vi "laneleftright412.vi"() -> (2 "Coeff right":dbl[](array[numeric]), 3 "Coeff left":dbl[](array[numeric]))   [LabVIEW 2015]
uses:
  <vilib>/Analysis/polynomials.llb/Remove Zero Threshold Type.ctl
  <vilib>/Analysis/1siggen.llb/Ramp Pattern by Samples.vi
  G_SEN.vi
  <vilib>/Analysis/1siggen.llb/Ramp Pattern by Delta.vi
  G_ALL.vi
  G_LCM.vi
  <vilib>/Analysis/polynomials.llb/1D Polynomial Evaluation (DBL).vi
  <vilib>/Analysis/polynomials.llb/Remove Zero Coefficients (DBL).vi
  <vilib>/Analysis/NI_AALPro.lvlib
  <vilib>/Analysis/NI_AALBase.lvlib
  <vilib>/Analysis/6fits.llb/Curve Fitting Criteria.ctl
panel:
  out "point_flag":i32[](array[numeric])
  out "gap":dbl
  out "residue":dbl
  out "appended array":dbl[](array[numeric])
  out "Steering coeff":dbl[](array[numeric])
  out "Coeff stop 2":dbl[](array[numeric])
  out "min value":dbl
  out "rin":dbl[](array[numeric])
  out "rout":dbl[](array[numeric])
  out "r":dbl[](array[numeric])
  out "wgain":dbl[](array[numeric])
  out "y 2":dbl[](array[numeric])
  out "x 2":dbl[](array[numeric])
  out "w 2":dbl[](array[numeric])
  out "lane_right_pt":dbl[][](array[numeric])
  in  "x_gain":dbl=1.0 min=-1.0 max=1.0
  in  "y_gain":dbl=1.0 min=-1.0 max=1.0
  out "map_track 2":dbl[][](array[numeric])
  in  "d_safe":dbl=1.1 format="%#_13g"
  out "map_track":dbl[][](array[numeric])
  out "lane_left_pt":dbl[][](array[numeric])
  out "x_shift":dbl format="%#_13g"
  out "y_shift":dbl format="%#_13g"
  in  "lane_gain":dbl=0.7 min=-1.0 max=1.0
  out "Lane_C_M":dbl[](array[numeric])=[0.8601491478953653, 0.8717844136967624, 0.882947592858927, 0.8936326403234123, 0.9038337699485205, 0.9135454576426009, 0.9227624443554423, 0.9314797389261423, 0.9396926207859084, 0.9473966425143293, 0.9545876322477319, 0.9612616959383189, 0.9674152194628639, 0.9730448705798238, 0.9781476007338057, 0.9827206467064133, 0.9867615321125792, 0.9902680687415704, 0.993238357741943, 0.9956707906498045, 0.9975640502598242, 0.9989171113385246, 0.9997292411794617, 1.0, 0.9997292411794617, 0.9989171113385246, 0.9975640502598242, 0.9956707906498045, 0.993238357741943, 0.9902680687415704, 0.9867615321125792, 0.9827206467064133]
  out "ratio(-1:left1:right)":dbl
  out "NaN/Path/Refnum?":bool
  out "Rleft":dbl
  out "Rright":dbl
  out "poly":i32=2 min=1 max=5 step=1
  out "y_end":dbl[](array[numeric])=[0.8601491478953653, 0.8717844136967624, 0.882947592858927, 0.8936326403234123, 0.9038337699485205, 0.9135454576426009, 0.9227624443554423, 0.9314797389261423, 0.9396926207859084, 0.9473966425143293, 0.9545876322477319, 0.9612616959383189, 0.9674152194628639, 0.9730448705798238, 0.9781476007338057, 0.9827206467064133, 0.9867615321125792, 0.9902680687415704, 0.993238357741943, 0.9956707906498045, 0.9975640502598242, 0.9989171113385246, 0.9997292411794617, 1.0, 0.9997292411794617, 0.9989171113385246, 0.9975640502598242, 0.9956707906498045, 0.993238357741943, 0.9902680687415704, 0.9867615321125792, 0.9827206467064133]
  in  "iter":i32=2
  out "Waveform Graph":dbl[](graph)
  out "w":dbl[](array[numeric])
  out "XY Graph 4":cluster{"Y":dbl[], "Y":dbl[]}[](graph)=[{"Y"=array[3210 elements], "Y"=array[3210 elements]}, {"Y"=[-0.0, 0.001154394197769193, 0.004617650635850623, 0.010389990872226917, 0.018471784248973222, 0.02886354801042046, 0.041565947468740205, 0.056579796217107514, 0.0739060563904701, 0.0935458389742223, 0.11550040416098284, 0.13977116175580306, 0.16635967162997645, 0.19526764422393228, 0.2264969410994837, 0.26004957554195585, 0.2959277132125635, 0.3341336728515216, 0.374669927032528, 0.417539102969144, 0.4627439833735707, 0.5102875073687159, 0.560172771454063, 0.6124030305261954, 0.6669816989546717, 0.7239123517142048, 0.7831987255740245, 0.8448447203451934, 0.9088544001870815, 0.975231994973953, 1.0439819017227023, 1.1151086860829622, 1.1886170838907617, 1.2645120027869723, 1.342798523901962, 1.42348190360768, 1.5065675753387922, 1.592061151484188, 1.6799684253507792, 1.770295373200753, 1.8630481563645134, 1.9582331234307588, 2.0558568125157564, 2.1559259536137603, 2.258447471030621], "Y"=[0.0, 0.5, 1.0, 1.5, 2.0, 2.5, 3.0, 3.5, 4.0, 4.5, 5.0, 5.5, 6.0, 6.5, 7.0, 7.5, 8.0, 8.5, 9.0, 9.5, 10.0, 10.5, 11.0, 11.5, 12.0, 12.5, 13.0, 13.5, 14.0, 14.5, 15.0, 15.5, 16.0, 16.5, 17.0, 17.5, 18.0, 18.5, 19.0, 19.5, 20.0, 20.5, 21.0, 21.5, 22.0]}, {"Y"=[0.362252581831572], "Y"=[-0.8199241909738847]}, {"Y"=array[210 elements], "Y"=array[210 elements]}, {"Y"=[-0.925, -0.925, -0.925, -0.6775, -0.6775, -0.925, -0.925, -0.925, -0.925, -0.6775, -0.6775, -0.925, -0.925, -0.925, 0.9025, 0.9025, 0.9025, 0.6775, 0.6775, 0.9025, 0.9025, 0.9025, 0.9025, 0.6775, 0.6775, 0.9025, 0.9025, 0.9025, -0.925], "Y"=[-0.75, -0.224, 0.224, 0.224, -0.224, -0.224, 0.224, 2.415, 2.885, 2.885, 2.415, 2.415, 2.885, 3.5, 3.5, 2.885, 2.415, 2.415, 2.885, 2.885, 2.415, 0.224, -0.224, -0.224, 0.224, 0.224, -0.224, -0.75, -0.75]}, {"Y"=[0.171875, 0.15377271904051304, 0.1346290179491043, 0.11445423440635205, 0.09325870609283447, 0.07105277068912982, 0.04784676587581635, 0.02365102933347224, -0.0015241012573242174, -0.02766828821599482, -0.05477119386196136, -0.08282248051464558, -0.11181181049346922, -0.14172884611785413, -0.17256324970722198, -0.20430468358099463, -0.23694281005859374, -0.27046729145944115, -0.30486779010295867, -0.340133968308568, -0.3762554883956909, -0.41322201268374914, -0.4510232034921646, -0.4896487231403589], "Y"=[0.0, 0.5, 1.0, 1.5, 2.0, 2.5, 3.0, 3.5, 4.0, 4.5, 5.0, 5.5, 6.0, 6.5, 7.0, 7.5, 8.0, 8.5, 9.0, 9.5, 10.0, 10.5, 11.0, 11.5]}, {"Y"=[1.796875, 1.778772719040513, 1.7596290179491043, 1.739454234406352, 1.7182587060928345, 1.6960527706891297, 1.6728467658758164, 1.6486510293334722, 1.6234758987426758, 1.5973317117840051, 1.5702288061380387, 1.5421775194853544, 1.513188189506531, 1.483271153882146, 1.452436750292778, 1.4206953164190055, 1.3880571899414063, 1.354532708540559, 1.3201322098970414, 1.284866031691432, 1.248744511604309, 1.2117779873162509, 1.1739767965078354, 1.135351276859641, 1.0959117660522462, 1.0556686017662287, 1.014632121682167, 0.9728126634806396, 0.9302205648422242, 0.8868661634474992], "Y"=[0.0, 0.5, 1.0, 1.5, 2.0, 2.5, 3.0, 3.5, 4.0, 4.5, 5.0, 5.5, 6.0, 6.5, 7.0, 7.5, 8.0, 8.5, 9.0, 9.5, 10.0, 10.5, 11.0, 11.5, 12.0, 12.5, 13.0, 13.5, 14.0, 14.5]}, {"Y"=[-1.453125, -1.471227280959487, -1.4903709820508957, -1.510545765593648, -1.5317412939071655, -1.5539472293108703, -1.5771532341241836, -1.6013489706665278, -1.6265241012573242, -1.6526682882159949, -1.6797711938619613, -1.7078224805146456, -1.736811810493469, -1.766728846117854, -1.797563249707222, -1.8293046835809945, -1.8619428100585937, -1.895467291459441, -1.9298677901029586], "Y"=[0.0, 0.5, 1.0, 1.5, 2.0, 2.5, 3.0, 3.5, 4.0, 4.5, 5.0, 5.5, 6.0, 6.5, 7.0, 7.5, 8.0, 8.5, 9.0]}, {"Y"=[0.171875, 0.2568230007600336, 0.3384052130063493, 0.44574342526006827, 0.5205081969556753, 0.5917680690742042, 0.659409530134929, 0.7229937549325056, 0.7835496148685115, 0.8405449546633443, 0.9258576868463875], "Y"=[-20.239964538708662, -19.725637940364884, -19.211158961966362, -18.6998967366845, -18.19022720070031, -17.681887266143153, -17.17615515566314, -16.67683575591291, -16.176265245349786, -15.679082775270938, -15.183754484614711]}, {"Y"=[7.134647485270904], "Y"=[38.71960961082238]}, {"Y"=array[980 elements], "Y"=array[980 elements]}, {"Y"=[], "Y"=[]}]
  out "y":dbl[](array[numeric])
  out "x":dbl[](array[numeric])
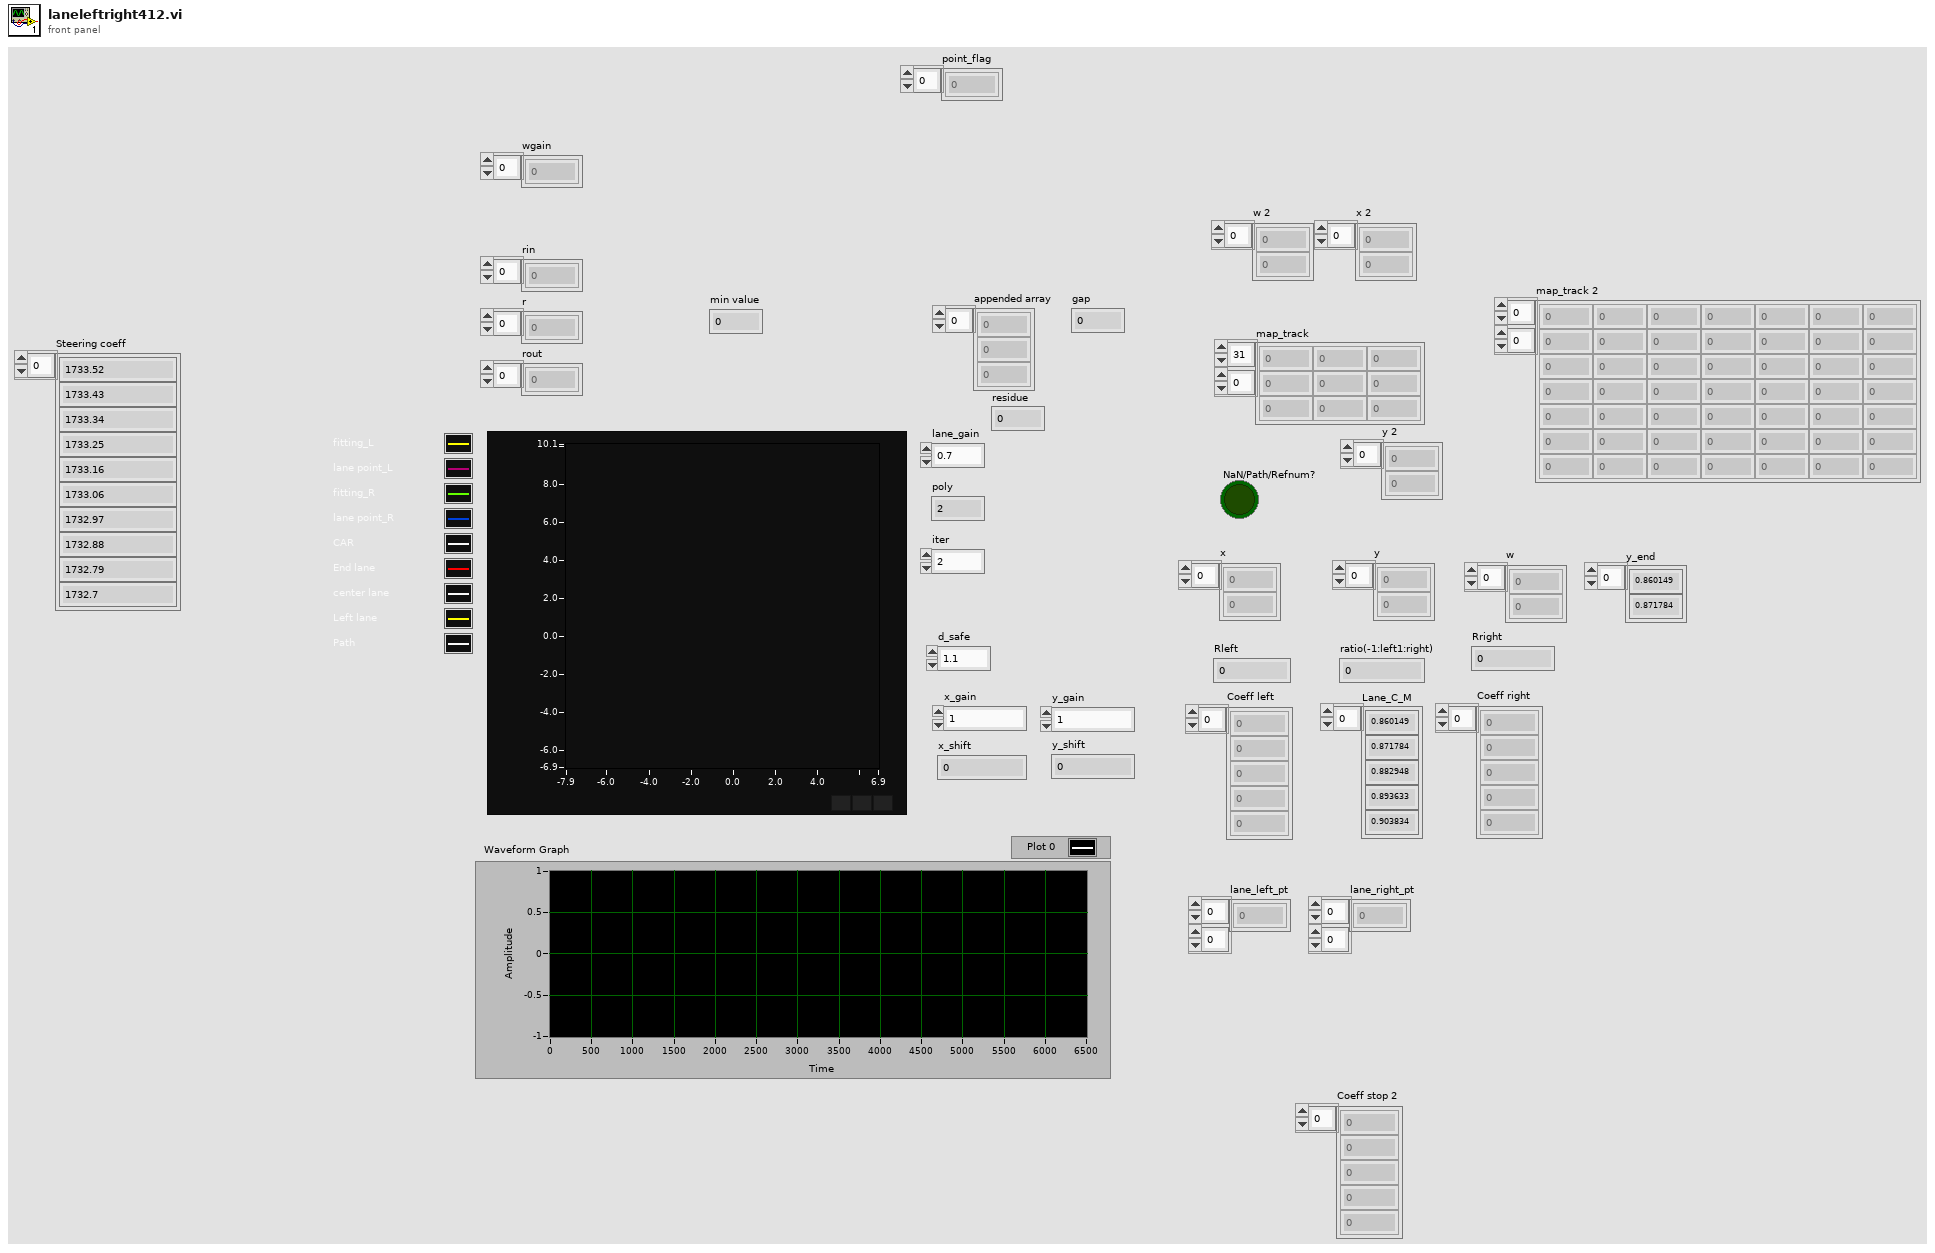
[diagram p1: front panel]
types:
  T1 = cluster{"C_Wheel base":dbl, "ratio_steer":dbl, "Overall width":dbl, "af":dbl, "turn radius":dbl, "eval":dbl, "ap":dbl, "an":dbl, "Vmax":dbl, "mu":dbl, "Vlast":dbl}
  T2 = cluster{"hash":i64, "sys time":i64, "size":i64, "x":dbl[], "y":dbl[], "point_flag":i32[]}
  T3 = cluster{"delta":bool, "Rotational position":dbl, "Rotational position":dbl, "Numeric":i32}[]
  T4 = cluster{"Steer_input":dbl, "Steer_output":dbl, "VS_des":dbl, "VS_can":dbl, "heading":dbl, "auto":bool, "run":bool, "x":dbl, "y":dbl, "slam_y":dbl, "slam_x":dbl, "slam_heading":dbl}
  T5 = typedef "NI_AALPro.lvlib/Curve Fitting Criteria.ctl" = u16
  T6 = typedef "NI_AALPro.lvlib/Remove Zero Threshold Type.ctl" = u16
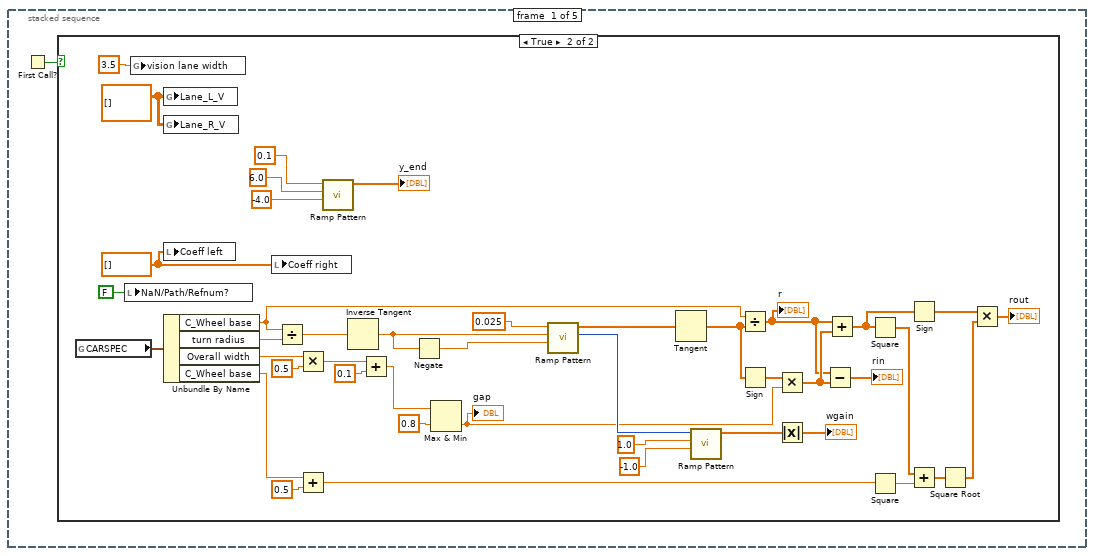
[diagram p2: hidden frame]
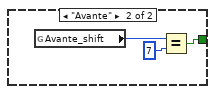
[diagram p5: hidden frame]
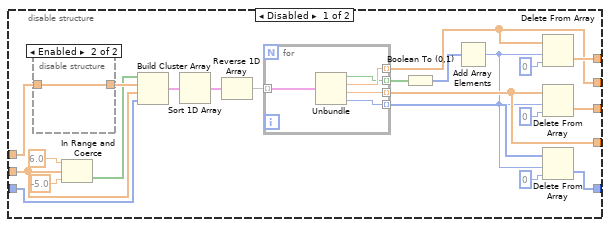
[diagram p6: hidden frame]
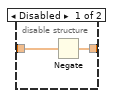
[diagram p7: hidden frame]
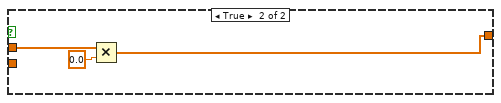
[diagram p8: hidden frame]
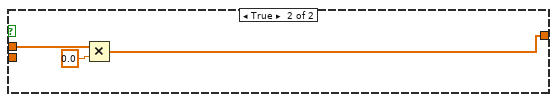
[diagram p9: hidden frame]
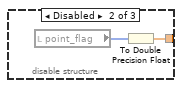
[diagram p10: hidden frame]
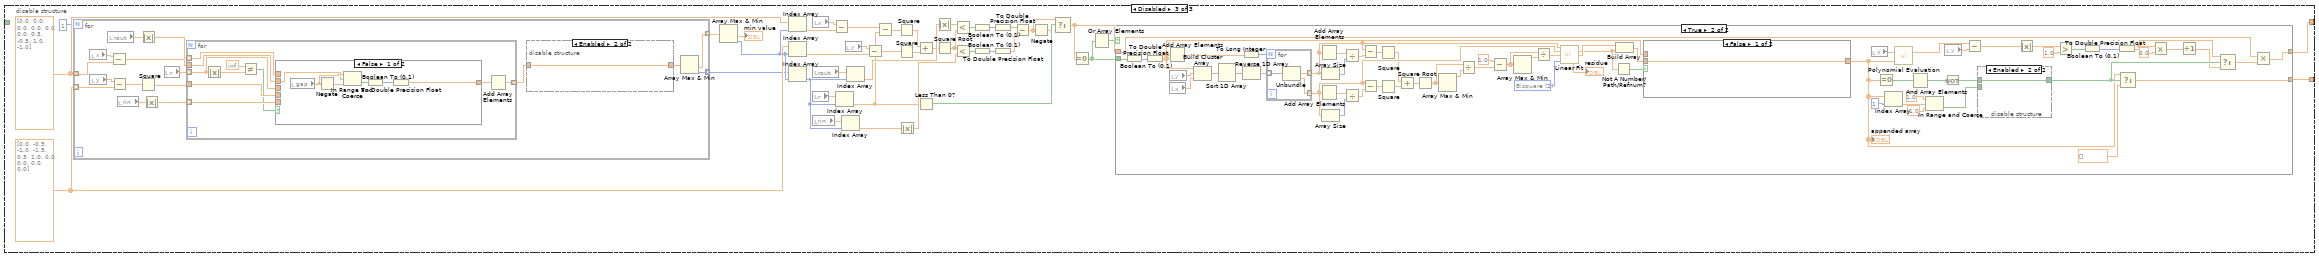
[diagram p11: hidden frame]
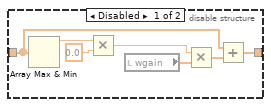
[diagram p12: hidden frame]
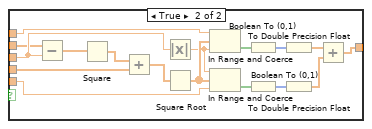
[diagram p13: hidden frame]
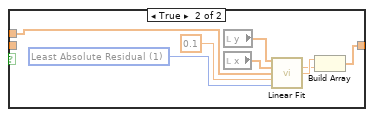
[diagram p15: hidden frame]
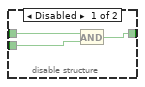
[diagram p16: hidden frame]
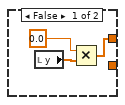
[diagram p17: hidden frame]
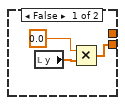
[diagram p18: hidden frame]
diagram:
  n1 = stacked-sequence {
    frame #0 {
      n2 = First Call?() -> (First Call?: T/F=w1:bool)
      n3 = case shown="True" w1 {
        frame False {
        }
        frame True {
          w37 = dbl[] [] ("Coeff left")
          w39 = dbl[][] [] ("Lane_R_V")
          n4 = global read "G_ALL.vi" "CARSPEC"() -> (w10:T1)
          n5 = local write "NaN/Path/Refnum?"(FALSE ("NaN/Path/Refnum?")) -> ()
          n6 = global write "G_SEN.vi" "vision lane width"(3.5 ("vision lane width")) -> ()
          n7 = global write "G_SEN.vi" "Lane_L_V"(w39) -> ()
          n8 = global write "G_SEN.vi" "Lane_R_V"(w39) -> ()
          n9 = local write "Coeff left"(w37) -> ()
          n10 = Unbundle By Name(w10) -> ("C_Wheel base"=w17:dbl, "turn radius"=w11:dbl, "Overall width"=w18:dbl, "C_Wheel base"=w3:dbl)
          n11 = local write "Coeff right"(w37) -> ()
          n12 = Divide(x=w17, y=w11) -> (x/y=w12:dbl)
          n13 = Multiply(x=w18, y=0.5) -> (x*y=w9:dbl)
          n14 = Add(x=w3, y=0.5) -> (x+y=w2:dbl)
          n15 = call-poly <vilib>:"Ramp Pattern.vi"("start"=-4.0, "end"=6.0, "delta"=0.1) -> ("Ramp Pattern"=→"y_end":dbl[])  [unwired: 6 in, 2 out]
          n16 = Inverse Tangent(1:w12) -> (0:w14:dbl)
          n17 = Add(x=w9, y=0.1) -> (x+y=w6:dbl)
          n18 = Negate(x=w14) -> (-x=w13:dbl)
          n19 = Max & Min(x=w6, y=0.8) -> (min(x,y)=w5:dbl)  [unwired: 1 out]
          "gap" <- w5
          n20 = call-poly <vilib>:"Ramp Pattern.vi"("start"=w13, "end"=w14, "delta"=0.025) -> ("samples"=w32:i32, "Ramp Pattern"=w16:dbl[])  [unwired: 6 in, 1 out]
          n21 = Tangent(1:w16) -> (0:w20:dbl[])
          n22 = call-poly <vilib>:"Ramp Pattern.vi"("start"=-1.0, "end"=1.0, "samples"=w32) -> ("Ramp Pattern"=w35:dbl[])  [unwired: 7 in, 1 out]
          n23 = Divide(x=w17, y=w20) -> (x/y=w23:dbl[])
          "r" <- w23
          n24 = Sign(1:w20) -> (0:w21:dbl[])
          n25 = Multiply(x=w21, y=w5) -> (x*y=w24:dbl[])
          n26 = Absolute Value(x=w35) -> (abs(x)=→"wgain":dbl[])
          n27 = Subtract(x=w23, y=w24) -> (x-y=→"rin":dbl[])
          n28 = Add(x=w23, y=w24) -> (x+y=w28:dbl[])
          n29 = Square(x=w28) -> (x^2=w25:dbl[])
          n30 = Square(x=w2) -> (x^2=w26:dbl)
          n31 = Sign(1:w28) -> (0:w30:dbl[])
          n32 = Add(x=w25, y=w26) -> (x+y=w27:dbl[])
          n33 = Square Root(x=w27) -> (sqrt(x)=w29:dbl[])
          n34 = Multiply(x=w30, y=w29) -> (x*y=→"rout":dbl[])
        }
      }
    }
    frame #1 {
      n35 = flat-sequence {
        tunnel: [w48] -> w45
        tunnel: w45 -> [w97]
        frame #0 {
          n36 = global read "G_LCM.vi" "VISION_LANE_PT"() -> (w52:T2)
          n37 = Unbundle By Name(w52) -> ("x"=w56:dbl[], "y"=w53:dbl[], "point_flag"=w46:i32[])
          n38 = disable-structure shown="Enabled" {
            disable-tunnel: w56 -> [w83 w95]
            disable-tunnel: [w81 w94] -> w55
            disable-tunnel: [w80 w95] -> w54
            disable-tunnel: w53 -> [w78 w94]
            disable-tunnel: [w69 w95] -> w51
            disable-tunnel: [w68 w94] -> w50
            disable-tunnel: [w63 w93] -> w47
            disable-tunnel: w46 -> [w67 w93]
            frame Disabled {
              n39 = disable-structure shown="Enabled" {
                disable-tunnel: w83 -> [w86 w87]
                disable-tunnel: [w85 w87] -> w84
                frame Disabled {
                  n40 = Negate(x=w86) -> (-x=w85:dbl[])
                }
                frame Enabled {
                }
              }
              n41 = In Range and Coerce(upper limit=6.0 ("delta"), x=w78, lower limit=-5.0) -> (In Range?=w76:bool[])  [unwired: 1 out]
              n42 = Build Cluster Array(w76, w84, w78, w67) -> (w74:T3)
              n43 = Sort 1D Array(array=w74) -> (sorted array=w75:T3)
              n44 = Reverse 1D Array(array=w75) -> (reversed array=w71:T3)
              n45 = for {
                tunnel: w71 -> [w92] mode=indexing
                tunnel: [w91] -> w69 mode=indexing
                tunnel: [w90] -> w68 mode=indexing
                tunnel: [w89] -> w79 mode=indexing
                tunnel: [w88] -> w66 mode=indexing
                n46 = Unbundle(w92) -> ("delta"=w89:bool, "Rotational position"=w91:dbl, "Rotational position"=w90:dbl, "Numeric"=w88:i32)
              }
              n47 = Boolean To (0,1)(Boolean=w79) -> (0, 1=w72:i16[])
              n48 = Add Array Elements(numeric array=w72) -> (sum=w65:i16)
              n49 = Delete From Array(array=w69, length=w65, index=0) -> (deleted portion=w80:dbl[])  [unwired: 1 out]
              n50 = Delete From Array(array=w68, length=w65, index=0) -> (deleted portion=w81:dbl[])  [unwired: 1 out]
              n51 = Delete From Array(array=w66, length=w65, index=0) -> (deleted portion=w63:i32[])  [unwired: 1 out]
            }
            frame Enabled {
            }
          }
          "x" <- w54
          "y" <- w55
          "x 2" <- w51
          "y 2" <- w50
          "point_flag" <- w47
          n52 = global read "G_LCM.vi" "car name"() -> (w49:string)
          n53 = case shown="Default" w49 {
            tunnel: [w57 w60] -> w48
            frame Default {
              n54 = global read "G_ALL.vi" "CARDATA"() -> (w59:T4)
              n55 = Unbundle By Name(w59) -> ("VS_can"=w58:dbl)
              n56 = Less Than 0?(x=w58) -> (x < 0?=w57:bool)
            }
            frame "Avante" {
              n57 = global read "G_ALL.vi" "Avante_shift"() -> (w62:u8)
              n58 = Equal?(x=w62, y=u8 7) -> (x = y?=w60:bool)
            }
          }
        }
        frame #1 {
          n59 = disable-structure shown="Enabled" {
            disable-tunnel: [w101 w163 w205] -> w96
            disable-tunnel: [_ _ w204] -> w98
            disable-tunnel: w97 -> [_ _ _]
            frame Enabled {
              n60 = local read "Coeff left"() -> (w130:dbl[])
              n61 = local read "Coeff right"() -> (w129:dbl[])
              n62 = Empty Array?(array=w130) -> (empty?=w131:bool)
              n63 = Empty Array?(array=w129) -> (empty?=w132:bool)
              n64 = local read "y"() -> (w127:dbl[])
              n65 = local read "x"() -> (w99:dbl[])
              n66 = local read "y"() -> (w133:dbl[])
              n67 = case shown="False" w131 {
                tunnel: w127 -> [w153 w161]
                tunnel: w130 -> [w150 _]
                tunnel: [w148 w160] -> w128
                frame False {
                  n68 = call-poly <vilib>:"Polynomial Evaluation.vi"("P(x)"=w150, "A"=w153) -> ("P(A)"=w152:dbl[])  [unwired: 1 out]
                  n69 = local read "x"() -> (w151:dbl[])
                  n70 = Subtract(x=w152, y=w151) -> (x-y=w157:dbl[])
                  n71 = Absolute Value(x=w157) -> (abs(x)=w156:dbl[])
                  n72 = Negate(x=w156) -> (-x=w155:dbl[])
                  n73 = Add(x=w155, y=1.0) -> (x+y=w159:dbl[])
                  n74 = Max & Min(x=0.0, y=w159) -> (max(x,y)=w149:dbl[])  [unwired: 1 out]
                  n75 = Negate(x=w149) -> (-x=w148:dbl[])
                }
                frame True {
                  n76 = Multiply(x=w161, y=0.0) -> (x*y=w160:dbl[])
                }
              }
              n77 = local read "y"() -> (w100:dbl[])
              n78 = case shown="False" w132 {
                tunnel: [w142 w145] -> w125
                tunnel: w129 -> [w141 _]
                tunnel: w133 -> [w134 w146]
                frame False {
                  n79 = call-poly <vilib>:"Polynomial Evaluation.vi"("P(x)"=w141, "A"=w134) -> ("P(A)"=w139:dbl[])  [unwired: 1 out]
                  n80 = local read "x"() -> (w140:dbl[])
                  n81 = Subtract(x=w139, y=w140) -> (x-y=w135:dbl[])
                  n82 = Absolute Value(x=w135) -> (abs(x)=w136:dbl[])
                  n83 = Negate(x=w136) -> (-x=w137:dbl[])
                  n84 = Add(x=w137, y=1.0) -> (x+y=w143:dbl[])
                  n85 = Max & Min(x=0.0, y=w143) -> (max(x,y)=w142:dbl[])  [unwired: 1 out]
                }
                frame True {
                  n86 = Multiply(x=w146, y=0.0) -> (x*y=w145:dbl[])
                }
              }
              n87 = Subtract(x=w99, y=6.0) -> (x-y=w103:dbl[])
              n88 = Subtract(x=w100, y=0.0) -> (x-y=w112:dbl[])
              n89 = Subtract(x=w99, y=-6.0) -> (x-y=w105:dbl[])
              n90 = Square(x=w105) -> (x^2=w104:dbl[])
              n91 = Square(x=w103) -> (x^2=w113:dbl[])
              n92 = Square(x=w112) -> (x^2=w114:dbl[])
              n93 = Add(x=w104, y=w114) -> (x+y=w120:dbl[])
              n94 = Add(x=w114, y=w113) -> (x+y=w115:dbl[])
              n95 = In Range and Coerce(upper limit=36.0, x=w120, lower limit=4.0) -> (In Range?=w122:bool[])  [unwired: 1 out]
              n96 = In Range and Coerce(upper limit=36.0, x=w115, lower limit=4.0) -> (In Range?=w121:bool[])  [unwired: 1 out]
              n97 = Boolean To (0,1)(Boolean=w122) -> (0, 1=w123:i16[])
              n98 = Boolean To (0,1)(Boolean=w121) -> (0, 1=w124:i16[])
              n99 = Multiply(x=i16 -1, y=w123) -> (x*y=w108:i16[])
              n100 = Add(x=w108, y=w124) -> (x+y=w110:i16[])
              n101 = Multiply(x=w110, y=1.0 ("element")) -> (x*y=w126:dbl[])
              n102 = Compound Arithmetic op=ADD(w126, w125, w128) -> (w101:dbl[])
            }
            frame Disabled {
              n103 = local read "point_flag"() -> (w164:i32[])
              n104 = To Double Precision Float(number=w164) -> (double precision float=w163:dbl[])
            }
            frame Disabled {
              w171 = dbl[] [0.0, -0.5, -1.0, -1.5, 0.5, 1.0, 0.0, 0.0, 0.0, 0.0]
              w169 = dbl[] [0.0, 0.0, 0.0, 0.0, 0.0, 0.0, 0.5, -0.5, 1.0, -1.0]
              n105 = for {
                N: 1 -> [_]
                tunnel: [w206] -> w166 mode=indexing
                tunnel: w169 -> [w211] mode=indexing
                tunnel: w171 -> [w209] mode=indexing
                tunnel: [w208] -> w167 mode=indexing
                n106 = local read "x"() -> (w213:dbl[])
                n107 = local read "y"() -> (w210:dbl[])
                n108 = local read "rout"() -> (w219:dbl[])
                n109 = Subtract(x=w213, y=w211) -> (x-y=w212:dbl[])
                n110 = Subtract(x=w210, y=w209) -> (x-y=w207:dbl[])
                n111 = local read "rin"() -> (w217:dbl[])
                n112 = Square(x=w207) -> (x^2=w220:dbl[])
                n113 = Absolute Value(x=w219) -> (abs(x)=w218:dbl[])
                n114 = Absolute Value(x=w217) -> (abs(x)=w216:dbl[])
                n115 = local read "r"() -> (w221:dbl[])
                n116 = for {
                  tunnel: w221 -> [w231] mode=indexing
                  tunnel: w220 -> [w239]
                  tunnel: w218 -> [w238] mode=indexing
                  tunnel: w216 -> [w237] mode=indexing
                  tunnel: [w236] -> w214 mode=indexing
                  tunnel: w212 -> [w235]
                  n117 = Absolute Value(x=w231) -> (abs(x)=w233:dbl)
                  n118 = Not Equal?(x=inf, y=w233) -> (x != y?=w230:bool)
                  n119 = case shown="False" w230 {
                    tunnel: w239 -> [_ w260]
                    tunnel: w238 -> [_ w257]
                    tunnel: w237 -> [_ w256]
                    tunnel: w231 -> [_ w252]
                    tunnel: w235 -> [w241 w247]
                    tunnel: [w240 w246] -> w234
                    frame False {
                      n120 = local read "gap"() -> (w242:dbl)
                      n121 = Negate(x=w242) -> (-x=w243:dbl)
                      n122 = In Range and Coerce(upper limit=w242, x=w241, lower limit=w243) -> (In Range?=w245:bool[])  [unwired: 1 out]
                      n123 = Boolean To (0,1)(Boolean=w245) -> (0, 1=w244:i16[])
                      n124 = To Double Precision Float(number=w244) -> (double precision float=w240:dbl[])
                    }
                    frame True {
                      n125 = Subtract(x=w247, y=w252) -> (x-y=w262:dbl[])
                      n126 = Square(x=w262) -> (x^2=w261:dbl[])
                      n127 = Add(x=w261, y=w260) -> (x+y=w259:dbl[])
                      n128 = Absolute Value(x=w252) -> (abs(x)=w253:dbl)
                      n129 = Square Root(x=w259) -> (sqrt(x)=w258:dbl[])
                      n130 = In Range and Coerce(upper limit=w257, x=w258, lower limit=w253) -> (In Range?=w249:bool[])  [unwired: 1 out]
                      n131 = In Range and Coerce(upper limit=w253, x=w258, lower limit=w256) -> (In Range?=w248:bool[])  [unwired: 1 out]
                      n132 = Boolean To (0,1)(Boolean=w249) -> (0, 1=w255:i16[])
                      n133 = Boolean To (0,1)(Boolean=w248) -> (0, 1=w254:i16[])
                      n134 = To Double Precision Float(number=w255) -> (double precision float=w251:dbl[])
                      n135 = To Double Precision Float(number=w254) -> (double precision float=w250:dbl[])
                      n136 = Add(x=w251, y=w250) -> (x+y=w246:dbl[])
                    }
                  }
                  n137 = Add Array Elements(numeric array=w234) -> (sum=w236:dbl)
                }
                n138 = disable-structure shown="Enabled" {
                  disable-tunnel: [w228 w229] -> w215
                  disable-tunnel: w214 -> [w224 w229]
                  frame Disabled {
                    n139 = Array Max & Min(array=w224) -> (max value=w227:dbl)  [unwired: 3 out]
                    n140 = Multiply(x=w227, y=0.0) -> (x*y=w223:dbl)
                    n141 = local read "wgain"() -> (w222:dbl[])
                    n142 = Multiply(x=w223, y=w222) -> (x*y=w225:dbl[])
                    n143 = Add(x=w224, y=w225) -> (x+y=w228:dbl[])
                  }
                  frame Enabled {
                  }
                }
                n144 = Array Max & Min(array=w215) -> (min value=w206:dbl, min index (indices)=w208:i32)  [unwired: 2 out]
              }
              n145 = Array Max & Min(array=w166) -> (min value=→"min value":dbl, min index (indices)=w170:i32)  [unwired: 2 out]
              n146 = Index Array(array=w169, index=w170) -> (element=w173:dbl)
              n147 = Index Array(array=w171, index=w170) -> (element=w172:dbl)
              n148 = Index Array(array=w167, index=w170) -> (element=w174:i32)
              n149 = local read "x"() -> (w197:dbl[])
              n150 = local read "rout"() -> (w193:dbl[])
              n151 = local read "r"() -> (w191:dbl[])
              n152 = local read "rin"() -> (w186:dbl[])
              n153 = Subtract(x=w197, y=w173) -> (x-y=w198:dbl[])
              n154 = Index Array(array=w191, index=w174) -> (element=w178:dbl)
              n155 = Index Array(array=w186, index=w174) -> (element=w180:dbl)
              n156 = local read "y"() -> (w199:dbl[])
              n157 = Index Array(array=w193, index=w174) -> (element=w192:dbl)
              n158 = Subtract(x=w199, y=w172) -> (x-y=w200:dbl[])
              n159 = Subtract(x=w198, y=w178) -> (x-y=w190:dbl[])
              n160 = Square(x=w190) -> (x^2=w189:dbl[])
              n161 = Square(x=w200) -> (x^2=w188:dbl[])
              n162 = Absolute Value(x=w180) -> (abs(x)=w179:dbl)
              n163 = Add(x=w189, y=w188) -> (x+y=w187:dbl[])
              n164 = Less Than 0?(x=w178) -> (x < 0?=w177:bool)
              n165 = Absolute Value(x=w192) -> (abs(x)=w194:dbl)
              n166 = Square Root(x=w187) -> (sqrt(x)=w195:dbl[])
              n167 = Less?(x=w194, y=w195) -> (x < y?=w196:bool[])
              n168 = Less?(x=w195, y=w179) -> (x < y?=w185:bool[])
              n169 = Boolean To (0,1)(Boolean=w196) -> (0, 1=w182:i16[])
              n170 = Boolean To (0,1)(Boolean=w185) -> (0, 1=w184:i16[])
              n171 = To Double Precision Float(number=w182) -> (double precision float=w181:dbl[])
              n172 = To Double Precision Float(number=w184) -> (double precision float=w183:dbl[])
              n173 = Subtract(x=w181, y=w183) -> (x-y=w176:dbl[])
              n174 = Negate(x=w176) -> (-x=w175:dbl[])
              n175 = Select(t=w176, s=w177, f=w175) -> (s? t:f=w203:dbl[])
              n176 = Equal To 0?(x=w203) -> (x = 0?=w202:bool[])
              n177 = Or Array Elements(Boolean array=w202) -> (logical OR=w201:bool)
              n178 = case shown="True" w201 {
                tunnel: [w263 w306] -> w205
                tunnel: w203 -> [w263 w305]
                tunnel: w202 -> [_ w298]
                tunnel: [_ w297] -> w204
                frame False {
                }
                frame True {
                  w299 = T5 2 items=["Least Square", "Least Absolute Residual", "Bisquare"] ("method")
                  n179 = Boolean To (0,1)(Boolean=w298) -> (0, 1=w302:i16[])
                  n180 = To Double Precision Float(number=w302) -> (double precision float=w289:dbl[])
                  n181 = Add Array Elements(numeric array=w289) -> (sum=w288:dbl)
                  n182 = local read "y"() -> (w293:dbl[])
                  n183 = local read "x"() -> (w292:dbl[])
                  n184 = Build Cluster Array(w289, w293, w292) -> (w291:cluster{dbl, dbl, dbl}[])
                  n185 = Sort 1D Array(array=w291) -> (sorted array=w290:cluster{dbl, dbl, dbl}[])
                  n186 = To Long Integer(number=w288) -> (32bit integer=w287:i32)
                  n187 = Reverse 1D Array(array=w290) -> (reversed array=w286:cluster{dbl, dbl, dbl}[])
                  n188 = for {
                    N: w287 -> [_]
                    tunnel: w286 -> [w329] mode=indexing
                    tunnel: [w328] -> w278 mode=indexing
                    tunnel: [w327] -> w276 mode=indexing
                    n189 = Unbundle(w329) -> (w328:dbl, w327:dbl)  [unwired: 1 out]
                  }
                  n190 = Add Array Elements(numeric array=w278) -> (sum=w282:dbl)
                  n191 = Add Array Elements(numeric array=w276) -> (sum=w281:dbl)
                  n192 = Array Size(array=w278) -> (size(s)=w283:i32)
                  n193 = Array Size(array=w276) -> (size(s)=w280:i32)
                  n194 = Divide(x=w282, y=w283) -> (x/y=w279:dbl)
                  n195 = Divide(x=w281, y=w280) -> (x/y=w277:dbl)
                  n196 = Subtract(x=w278, y=w279) -> (x-y=w275:dbl[])
                  n197 = Subtract(x=w276, y=w277) -> (x-y=w274:dbl[])
                  n198 = Square(x=w275) -> (x^2=w272:dbl[])
                  n199 = Square(x=w274) -> (x^2=w273:dbl[])
                  n200 = Add(x=w272, y=w273) -> (x+y=w271:dbl[])
                  n201 = Square Root(x=w271) -> (sqrt(x)=w269:dbl[])
                  n202 = Array Max & Min(array=w269) -> (max value=w270:dbl)  [unwired: 3 out]
                  n203 = Divide(x=w269, y=w270) -> (x/y=w268:dbl[])
                  n204 = Subtract(x=1.0, y=w268) -> (x-y=w265:dbl[])
                  n205 = Array Max & Min(array=w265) -> (max value=w266:dbl)  [unwired: 3 out]
                  n206 = Divide(x=w265, y=w266) -> (x/y=w264:dbl[])
                  n207 = call <vilib>:"Linear Fit.vi"("Y"=w278, "X"=w276, "Weight"=w264, "method"=w299) -> ("slope"=w296:dbl, "intercept"=w300:dbl, "residue"=→"residue":dbl)  [unwired: 7 in, 2 out]
                  n208 = Not A Number/Path/Refnum?(number/path/refnum=w296) -> (NaN/Path/Refnum?=w285:bool)
                  n209 = Build Array(w300, w296) -> (w294:dbl[])
                  n210 = case shown="False" w285 {
                    tunnel: w289 -> [_ w336]
                    tunnel: [w330 w333] -> w295
                    tunnel: w294 -> [w330 _]
                    frame False {
                    }
                    frame True {
                      w338 = T5 1 items=["Least Square", "Least Absolute Residual", "Bisquare"] ("method")
                      n211 = local read "y"() -> (w332:dbl[])
                      n212 = local read "x"() -> (w331:dbl[])
                      n213 = call <vilib>:"Linear Fit.vi"("Y"=w332, "X"=w331, "Weight"=w336, "tolerance"=0.1, "method"=w338) -> ("slope"=w334:dbl, "intercept"=w335:dbl)  [unwired: 6 in, 3 out]
                      n214 = Build Array(w335, w334) -> (w333:dbl[])
                    }
                  }
                  "appended array" <- w295
                  n215 = local read "x"() -> (w307:dbl[])
                  n216 = Equal To 0?(x=w295) -> (x = 0?=w321:bool[])
                  n217 = Index Array(array=w295, index=1) -> (element=w314:dbl)
                  n218 = call-poly <vilib>:"Polynomial Evaluation.vi"("P(x)"=w295, "A"=w307) -> ("P(A)"=w308:dbl[])  [unwired: 1 out]
                  n219 = And Array Elements(Boolean array=w321) -> (logical AND=w324:bool)
                  n220 = In Range and Coerce(upper limit=1.0, x=w314, lower limit=-1.0) -> (In Range?=w322:bool)  [unwired: 1 out]
                  n221 = Not(x=w324) -> (.not. x?=w325:bool)
                  n222 = local read "y"() -> (w309:dbl[])
                  n223 = Subtract(x=w308, y=w309) -> (x-y=w301:dbl[])
                  n224 = disable-structure shown="Enabled" {
                    disable-tunnel: w322 -> [w341 _]
                    disable-tunnel: [w340 w342] -> w323
                    disable-tunnel: w325 -> [w339 w342]
                    frame Disabled {
                      n225 = And(x=w339, y=w341) -> (x .and. y?=w340:bool)
                    }
                    frame Enabled {
                    }
                  }
                  n226 = Absolute Value(x=w301) -> (abs(x)=w310:dbl[])
                  n227 = Greater?(x=w310, y=1.0 ("Numeric 2")) -> (0:w312:bool[])
                  n228 = Boolean To (0,1)(Boolean=w312) -> (0, 1=w304:i16[])
                  n229 = To Double Precision Float(number=w304) -> (double precision float=w303:dbl[])
                  n230 = Select(t=w295, s=w323, f=dbl[] []) -> (s? t:f=w297:dbl[])
                  n231 = Multiply(x=w303, y=0.0) -> (x*y=w318:dbl[])
                  n232 = Increment(x=w318) -> (x+1=w319:dbl[])
                  n233 = Select(t=w303, s=w323, f=w319) -> (s? t:f=w326:dbl[])
                  n234 = Multiply(x=w305, y=w326) -> (x*y=w306:dbl[])
                }
              }
            }
          }
          "w" <- w96
          "Coeff stop 2" <- w98
        }
        frame #2 {
          n235 = local read "w"() -> (w356:dbl[])
          n236 = Not Equal To 0?(x=w356) -> (x != 0?=w349:bool[])
          n237 = local read "w"() -> (w355:dbl[])
          n238 = local read "x"() -> (w354:dbl[])
          n239 = local read "y"() -> (w353:dbl[])
          n240 = Boolean To (0,1)(Boolean=w349) -> (0, 1=w348:i16[])
          n241 = Build Cluster Array(w349, w355, w354, w353) -> (w352:cluster{bool, dbl, dbl, dbl}[])
          n242 = To Long Integer(number=w348) -> (32bit integer=w347:i32[])
          n243 = Sort 1D Array(array=w352) -> (sorted array=w351:cluster{bool, dbl, dbl, dbl}[])
          n244 = Add Array Elements(numeric array=w347) -> (sum=w346:i32)
          n245 = Reverse 1D Array(array=w351) -> (reversed array=w350:cluster{bool, dbl, dbl, dbl}[])
          n246 = for {
            N: w346 -> [_]
            tunnel: w350 -> [w360] mode=indexing
            tunnel: [w359] -> w343 mode=indexing
            tunnel: [w358] -> w345 mode=indexing
            tunnel: [w357] -> w344 mode=indexing
            n247 = Unbundle(w360) -> (w359:dbl, w358:dbl, w357:dbl)  [unwired: 1 out]
          }
          n248 = local write "w"(w343) -> ()
          n249 = local write "x"(w345) -> ()
          n250 = local write "y"(w344) -> ()
        }
        frame #3 {
          w363 = T6 0 items=["Absolute Value", "Relative Value"] ("threshold type")
          n251 = global read "G_ALL.vi" "Steering coeff"() -> (w364:dbl[])
          "Steering coeff" <- w364
          n252 = Empty Array?(array=w364) -> (empty?=w368:bool)
          n253 = Delete From Array(array=w364, index=0) -> (array with subset deleted=w366:dbl[])  [unwired: 1 in, 1 out]
          n254 = call-poly <vilib>:"Remove Zero Coefficients.vi"("threshold type"=w363, "threshold"=0.02, "P(x) In"=w366) -> ("P(x) Out"=w367:dbl[])  [unwired: 6 in, 2 out]
          n255 = Array Size(array=w367) -> (size(s)=w370:i32)
          n256 = Max & Min(x=w370, y=2) -> (min(x,y)=w371:i32)  [unwired: 1 out]
          n257 = Select(t=2, s=w368, f=w371) -> (s? t:f=→"poly":i32)
        }
        frame #4 {
          n258 = for {
            N: "iter" -> [_]
            n259 = flat-sequence {
              tunnel: [w420] -> w376
              tunnel: [w486] -> w375
              tunnel: w376 -> [w486]
              tunnel: [w485] -> w374
              tunnel: w375 -> [w511]
              tunnel: w374 -> [w510]
              frame #0 {
                n260 = local read "w"() -> (w379:dbl[])
                n261 = Equal?(x=w379, y=1.0) -> (x = y?=w378:bool[])
                n262 = Boolean To (0,1)(Boolean=w378) -> (0, 1=w414:i16[])
                n263 = To Double Precision Float(number=w414) -> (double precision float=w409:dbl[])
                n264 = Add Array Elements(numeric array=w409) -> (sum=w408:dbl)
                n265 = local read "x"() -> (w413:dbl[])
                n266 = local read "y"() -> (w412:dbl[])
                n267 = Build Cluster Array(w409, w413, w412) -> (w411:cluster{dbl, dbl, dbl}[])
                n268 = Sort 1D Array(array=w411) -> (sorted array=w410:cluster{dbl, dbl, dbl}[])
                n269 = To Long Integer(number=w408) -> (32bit integer=w407:i32)
                n270 = Reverse 1D Array(array=w410) -> (reversed array=w406:cluster{dbl, dbl, dbl}[])
                n271 = for {
                  N: w407 -> [_]
                  tunnel: w406 -> [w423] mode=indexing
                  tunnel: [w422] -> w392 mode=indexing
                  tunnel: [w421] -> w391 mode=indexing
                  n272 = Unbundle(w423) -> (w422:dbl, w421:dbl)  [unwired: 1 out]
                }
                n273 = Add Array Elements(numeric array=w392) -> (sum=w404:dbl)
                n274 = Add Array Elements(numeric array=w391) -> (sum=w403:dbl)
                n275 = Array Size(array=w392) -> (size(s)=w405:i32)
                n276 = Array Size(array=w391) -> (size(s)=w402:i32)
                n277 = Divide(x=w404, y=w405) -> (x/y=w401:dbl)
                n278 = Divide(x=w403, y=w402) -> (x/y=w400:dbl)
                n279 = Subtract(x=w392, y=w401) -> (x-y=w399:dbl[])
                n280 = Subtract(x=w391, y=w400) -> (x-y=w398:dbl[])
                n281 = Square(x=w399) -> (x^2=w396:dbl[])
                n282 = Square(x=w398) -> (x^2=w397:dbl[])
                n283 = Add(x=w396, y=w397) -> (x+y=w395:dbl[])
                n284 = Square Root(x=w395) -> (sqrt(x)=w394:dbl[])
                n285 = Array Max & Min(array=w394) -> (max value=w386:dbl)  [unwired: 3 out]
                n286 = Divide(x=w394, y=w386) -> (x/y=w393:dbl[])
                n287 = Multiply(x=w386, y=0.025) -> (x*y=w384:dbl)
                n288 = Subtract(x=1.0, y=w384) -> (x-y=w382:dbl)
                n289 = Max & Min(x=w382, y=0.5) -> (max(x,y)=w380:dbl)  [unwired: 1 out]
                n290 = Subtract(x=w380, y=w393) -> (x-y=w390:dbl[])
                n291 = Max & Min(x=w390, y=0.0) -> (max(x,y)=w388:dbl[])  [unwired: 1 out]
                n292 = Not Equal To 0?(x=w388) -> (x != 0?=w387:bool[])
                n293 = Boolean To (0,1)(Boolean=w387) -> (0, 1=w415:i16[])
                n294 = Add Array Elements(numeric array=w415) -> (sum=w418:i16)
                n295 = Greater?(x=w418, y=i16 50) -> (0:w416:bool)
                n296 = case shown="True" w416 {
                  tunnel: [w425 w432] -> w420
                  tunnel: [_ w431] -> w419
                  tunnel: w392 -> [_ w430]
                  tunnel: w391 -> [_ w429]
                  tunnel: w388 -> [_ w428]
                  frame False {
                    n297 = local read "y"() -> (w426:dbl[])
                    n298 = Multiply(x=0.0, y=w426) -> (x*y=w425:dbl[])
                  }
                  frame True {
                    n299 = local read "poly"() -> (w427:i32)
                    n300 = call <vilib>:"General Polynomial Fit Coefficients.vi"("Y"=w430, "polynomial order"=w427, "X"=w429, "Weight"=w428) -> ("Polynomial Coefficients"=w431:dbl[])  [unwired: 10 in, 1 out]
                    n301 = local read "y"() -> (w441:dbl[])
                    n302 = call-poly <vilib>:"Polynomial Evaluation.vi"("P(x)"=w431, "A"=w441) -> ("P(A)"=w440:dbl[])  [unwired: 1 out]
                    n303 = local read "x"() -> (w439:dbl[])
                    n304 = Subtract(x=w440, y=w439) -> (x-y=w438:dbl[])
                    n305 = Absolute Value(x=w438) -> (abs(x)=w437:dbl[])
                    n306 = Negate(x=w437) -> (-x=w436:dbl[])
                    n307 = Add(x=w436, y=1.0) -> (x+y=w433:dbl[])
                    n308 = Max & Min(x=0.0, y=w433) -> (max(x,y)=w432:dbl[])  [unwired: 1 out]
                  }
                }
                "Coeff right" <- w419
              }
              frame #1 {
                n309 = local read "w"() -> (w481:dbl[])
                n310 = Equal?(x=w481, y=-1.0) -> (x = y?=w482:bool[])
                n311 = Boolean To (0,1)(Boolean=w482) -> (0, 1=w449:i16[])
                n312 = To Double Precision Float(number=w449) -> (double precision float=w454:dbl[])
                n313 = Add Array Elements(numeric array=w454) -> (sum=w455:dbl)
                n314 = local read "x"() -> (w450:dbl[])
                n315 = local read "y"() -> (w451:dbl[])
                n316 = Build Cluster Array(w454, w450, w451) -> (w452:cluster{dbl, dbl, dbl}[])
                n317 = Sort 1D Array(array=w452) -> (sorted array=w453:cluster{dbl, dbl, dbl}[])
                n318 = To Long Integer(number=w455) -> (32bit integer=w456:i32)
                n319 = Reverse 1D Array(array=w453) -> (reversed array=w457:cluster{dbl, dbl, dbl}[])
                n320 = for {
                  N: w456 -> [_]
                  tunnel: w457 -> [w489] mode=indexing
                  tunnel: [w488] -> w445 mode=indexing
                  tunnel: [w487] -> w444 mode=indexing
                  n321 = Unbundle(w489) -> (w488:dbl, w487:dbl)  [unwired: 1 out]
                }
                n322 = Add Array Elements(numeric array=w445) -> (sum=w459:dbl)
                n323 = Add Array Elements(numeric array=w444) -> (sum=w460:dbl)
                n324 = Array Size(array=w445) -> (size(s)=w458:i32)
                n325 = Array Size(array=w444) -> (size(s)=w461:i32)
                n326 = Divide(x=w459, y=w458) -> (x/y=w462:dbl)
                n327 = Divide(x=w460, y=w461) -> (x/y=w463:dbl)
                n328 = Subtract(x=w445, y=w462) -> (x-y=w464:dbl[])
                n329 = Subtract(x=w444, y=w463) -> (x-y=w465:dbl[])
                n330 = Square(x=w464) -> (x^2=w467:dbl[])
                n331 = Square(x=w465) -> (x^2=w466:dbl[])
                n332 = Add(x=w467, y=w466) -> (x+y=w468:dbl[])
                n333 = Square Root(x=w468) -> (sqrt(x)=w469:dbl[])
                n334 = Array Max & Min(array=w469) -> (max value=w474:dbl)  [unwired: 3 out]
                n335 = Divide(x=w469, y=w474) -> (x/y=w470:dbl[])
                n336 = Multiply(x=w474, y=0.025) -> (x*y=w476:dbl)
                n337 = Subtract(x=1.0, y=w476) -> (x-y=w478:dbl)
                n338 = Max & Min(x=w478, y=0.5) -> (max(x,y)=w480:dbl)  [unwired: 1 out]
                n339 = Subtract(x=w480, y=w470) -> (x-y=w471:dbl[])
                n340 = Max & Min(x=w471, y=0.0) -> (max(x,y)=w443:dbl[])  [unwired: 1 out]
                n341 = Not Equal To 0?(x=w443) -> (x != 0?=w473:bool[])
                n342 = Boolean To (0,1)(Boolean=w473) -> (0, 1=w448:i16[])
                n343 = Add Array Elements(numeric array=w448) -> (sum=w446:i16)
                n344 = Greater?(x=w446, y=i16 50) -> (0:w442:bool)
                n345 = case shown="True" w442 {
                  tunnel: [w490 w498] -> w485
                  tunnel: [_ w497] -> w484
                  tunnel: w445 -> [_ w495]
                  tunnel: w444 -> [_ w494]
                  tunnel: w443 -> [_ w493]
                  frame False {
                    n346 = local read "y"() -> (w491:dbl[])
                    n347 = Multiply(x=0.0, y=w491) -> (x*y=w490:dbl[])
                  }
                  frame True {
                    n348 = local read "poly"() -> (w496:i32)
                    n349 = call <vilib>:"General Polynomial Fit Coefficients.vi"("Y"=w495, "polynomial order"=w496, "X"=w494, "Weight"=w493) -> ("Polynomial Coefficients"=w497:dbl[])  [unwired: 10 in, 1 out]
                    n350 = local read "y"() -> (w502:dbl[])
                    n351 = call-poly <vilib>:"Polynomial Evaluation.vi"("P(x)"=w497, "A"=w502) -> ("P(A)"=w503:dbl[])  [unwired: 1 out]
                    n352 = local read "x"() -> (w504:dbl[])
                    n353 = Subtract(x=w503, y=w504) -> (x-y=w505:dbl[])
                    n354 = Absolute Value(x=w505) -> (abs(x)=w506:dbl[])
                    n355 = Negate(x=w506) -> (-x=w500:dbl[])
                    n356 = Add(x=w500, y=1.0) -> (x+y=w507:dbl[])
                    n357 = Max & Min(x=0.0, y=w507) -> (max(x,y)=w501:dbl[])  [unwired: 1 out]
                    n358 = Negate(x=w501) -> (-x=w498:dbl[])
                  }
                }
                "Coeff left" <- w484
              }
              frame #2 {
                n359 = local read "w"() -> (w515:dbl[])
                n360 = disable-structure shown="Enabled" {
                  disable-tunnel: w515 -> [w519 w520]
                  disable-tunnel: w511 -> [w518 _]
                  disable-tunnel: [w517 w520] -> w509
                  disable-tunnel: w510 -> [w516 _]
                  frame Enabled {
                    n361 = Compound Arithmetic op=ADD(w516, w519, w518) -> (w517:dbl[])
                  }
                  frame Disabled {
                  }
                }
                n362 = In Range and Coerce(upper limit=1.0, x=w509, lower limit=-1.0) -> (coerced(x)=w512:dbl[])  [unwired: 1 out]
                n363 = disable-structure shown="Enabled" {
                  disable-tunnel: w512 -> [w521 _]
                  frame Enabled {
                    n364 = local write "w"(w521) -> ()
                  }
                  frame Disabled {
                  }
                }
              }
            }
          }
        }
        frame #5 {
          n365 = disable-structure shown="Enabled" {
            disable-tunnel: [w532 _] -> w522
            frame Enabled {
              n366 = local read "Coeff left"() -> (w531:dbl[])
              n367 = Index Array(array=w531, index=1) -> (element=w534:dbl)
              n368 = Absolute Value(x=w534) -> (abs(x)=w535:dbl)
              n369 = Less?(x=w535, y=1.0) -> (x < y?=w537:bool)
              n370 = Select(t=w531, s=w537, f=dbl[] []) -> (s? t:f=w532:dbl[])
            }
            frame Disabled {
            }
          }
          n371 = disable-structure shown="Enabled" {
            frame Enabled {
              n372 = local read "Coeff right"() -> (w523:dbl[])
              n373 = Index Array(array=w523, index=1) -> (element=w528:dbl)
              n374 = Absolute Value(x=w528) -> (abs(x)=w527:dbl)
              n375 = Less?(x=w527, y=1.0) -> (x < y?=w525:bool)
              n376 = Select(t=w523, s=w525, f=dbl[] []) -> (s? t:f=w530:dbl[])
              n377 = local write "Coeff right"(w530) -> ()
            }
            frame Disabled {
            }
          }
          n378 = local write "Coeff left"(w522) -> ()
        }
        frame #6 {
          n379 = local read "Coeff right"() -> (w540:dbl[])
          n380 = local read "Coeff left"() -> (w539:dbl[])
          n381 = Empty Array?(array=w539) -> (empty?=w543:bool)
          n382 = Empty Array?(array=w540) -> (empty?=w541:bool)
          n383 = Exclusive Or(1:w541, 2:w543) -> (0:w542:bool)
          n384 = case shown="True" w542 {
            tunnel: w543 -> [_ w563]
            frame False {
              n385 = local read "Coeff right"() -> (w547:dbl[])
              n386 = local read "Coeff left"() -> (w548:dbl[])
              n387 = Index Array(array=w548) -> (element=w546:dbl)  [unwired: 1 in]
              n388 = Index Array(array=w547) -> (element=w545:dbl)  [unwired: 1 in]
              n389 = Greater?(x=w546, y=w545) -> (0:w544:bool)
              n390 = case shown="True" w544 {
                frame False {
                }
                frame True {
                  n391 = flat-sequence {
                    tunnel: [w556] -> w552
                    tunnel: [w555] -> w551
                    tunnel: [w554] -> w550
                    tunnel: [w560] -> w553
                    tunnel: w552 -> [w560]
                    tunnel: w551 -> [w559]
                    tunnel: w550 -> [w558]
                    tunnel: [w557] -> w549
                    tunnel: w553 -> [w562]
                    tunnel: w549 -> [w561]
                    frame #0 {
                      n392 = local read "Coeff right"() -> (w556:dbl[])
                      n393 = local read "Coeff left"() -> (w555:dbl[])
                      n394 = local read "w"() -> (w554:dbl[])
                    }
                    frame #1 {
                      n395 = local write "Coeff right"(w559) -> ()
                      n396 = Negate(x=w558) -> (-x=w557:dbl[])
                    }
                    frame #2 {
                      n397 = local write "w"(w561) -> ()
                      n398 = local write "Coeff left"(w562) -> ()
                    }
                  }
                }
              }
            }
            frame True {
              n399 = case shown="True" w563 {
                frame False {
                  n400 = local read "Coeff left"() -> (w568:dbl[])
                  n401 = Index Array(array=w568, index=0) -> (element=w566:dbl)
                  n402 = Greater?(x=w566, y=0.5) -> (0:w564:bool)
                  n403 = case shown="True" w564 {
                    frame False {
                    }
                    frame True {
                      n404 = flat-sequence {
                        frame #0 {
                          n405 = local read "Coeff left"() -> (w571:dbl[])
                          n406 = local read "w"() -> (w570:dbl[])
                          n407 = Negate(x=w570) -> (-x=w569:dbl[])
                          n408 = local write "Coeff right"(w571) -> ()
                          n409 = local write "w"(w569) -> ()
                        }
                        frame #1 {
                          n410 = local write "Coeff left"(dbl[] []) -> ()
                        }
                      }
                    }
                  }
                }
                frame True {
                  n411 = local read "Coeff right"() -> (w577:dbl[])
                  n412 = Index Array(array=w577, index=0) -> (element=w575:dbl)
                  n413 = Less?(x=w575, y=-0.5) -> (x < y?=w573:bool)
                  n414 = case shown="True" w573 {
                    frame False {
                    }
                    frame True {
                      n415 = flat-sequence {
                        frame #0 {
                          n416 = local read "Coeff right"() -> (w580:dbl[])
                          n417 = local read "w"() -> (w579:dbl[])
                          n418 = Negate(x=w579) -> (-x=w578:dbl[])
                          n419 = local write "Coeff left"(w580) -> ()
                          n420 = local write "w"(w578) -> ()
                        }
                        frame #1 {
                          n421 = local write "Coeff right"(dbl[] []) -> ()
                        }
                      }
                    }
                  }
                }
              }
            }
          }
        }
        frame #7 {
          n422 = local read "Coeff right"() -> (w583:dbl[])
          n423 = local read "Coeff left"() -> (w582:dbl[])
          n424 = global write "G_SEN.vi" "Lane_L_M"(w582) -> ()
          n425 = global write "G_SEN.vi" "Lane_R_M"(w583) -> ()
        }
      }
    }
    frame #2 {
      n426 = flat-sequence {
        frame #0 {
          n427 = local read "Coeff right"() -> (w585:dbl[])
          n428 = local read "Coeff right"() -> (w613:dbl[])
          n429 = local read "Coeff left"() -> (w584:dbl[])
          n430 = local read "Coeff left"() -> (w611:dbl[])
          n431 = Empty Array?(array=w584) -> (empty?=w587:bool)
          n432 = Empty Array?(array=w585) -> (empty?=w588:bool)
          n433 = Empty Array?(array=w611) -> (empty?=w605:bool)
          n434 = Empty Array?(array=w613) -> (empty?=w607:bool)
          n435 = Index Array(array=w611, index #1=1 ("index")) -> (element #1=w604:dbl, element #2=w597:dbl)  [unwired: 1 in]
          n436 = Index Array(array=w613, index #1=1 ("index")) -> (element #1=w589:dbl, element #2=w596:dbl)  [unwired: 1 in]
          n437 = Square(x=w604) -> (x^2=w603:dbl)
          n438 = Square(x=w589) -> (x^2=w590:dbl)
          n439 = Or(x=w587, y=w588) -> (x .or. y?=w586:bool)
          n440 = case shown="False" w586 {
            frame False {
              n441 = local read "Coeff right"() -> (w620:dbl[])
              n442 = local read "Coeff left"() -> (w617:dbl[])
              n443 = Subtract(x=w620, y=w617) -> (x-y=w618:dbl[])
              n444 = Index Array(array=w618, index=0) -> (element=w621:dbl)
              n445 = Max & Min(x=w621, y=2.0) -> (max(x,y)=w622:dbl)  [unwired: 1 out]
              n446 = global write "G_SEN.vi" "vision lane width"(w622) -> ()
            }
            frame True {
            }
          }
          n447 = Increment(x=w603) -> (x+1=w601:dbl)
          n448 = Increment(x=w590) -> (x+1=w592:dbl)
          n449 = Multiply(x=w596, y=2.0) -> (x*y=w594:dbl)
          n450 = Square Root(x=w601) -> (sqrt(x)=w602:dbl)
          n451 = Square Root(x=w592) -> (sqrt(x)=w591:dbl)
          n452 = Multiply(x=w597, y=2.0) -> (x*y=w599:dbl)
          n453 = Multiply(x=w602, y=w601) -> (x*y=w600:dbl)
          n454 = Multiply(x=w591, y=w592) -> (x*y=w593:dbl)
          n455 = Divide(x=w600, y=w599) -> (x/y=w606:dbl)
          n456 = Divide(x=w593, y=w594) -> (x/y=w608:dbl)
          n457 = Select(t=inf, s=w605, f=w606) -> (s? t:f=→"Rleft":dbl)
          n458 = Select(t=inf, s=w607, f=w608) -> (s? t:f=→"Rright":dbl)
        }
        frame #1 {
          n459 = local read "Rright"() -> (w624:dbl)
          n460 = local read "Rleft"() -> (w625:dbl)
          n461 = disable-structure shown="Enabled" {
            disable-tunnel: w624 -> [w636 w646 _]
            disable-tunnel: w625 -> [w635 w645 _]
            disable-tunnel: [w632 w638 TRUE] -> w626
            frame Disabled {
              n462 = Sign(1:w636) -> (0:w634:dbl)
              n463 = Sign(1:w635) -> (0:w633:dbl)
              n464 = Equal?(x=w634, y=w633) -> (x = y?=w632:bool)
            }
            frame Enabled {
              w650 = inf
              n465 = Sign(1:w646) -> (0:w644:dbl)
              n466 = Sign(1:w645) -> (0:w643:dbl)
              n467 = Absolute Value(x=w646) -> (abs(x)=w651:dbl)
              n468 = Absolute Value(x=w645) -> (abs(x)=w649:dbl)
              n469 = Not Equal?(x=w644, y=w643) -> (x != y?=w641:bool)
              n470 = Not Equal?(x=w651, y=w650) -> (x != y?=w648:bool)
              n471 = Not Equal?(x=w650, y=w649) -> (x != y?=w647:bool)
              n472 = Or(x=w648, y=w647) -> (x .or. y?=w639:bool)
              n473 = And(x=w648, y=w647) -> (x .and. y?=w642:bool)
              n474 = And(x=w642, y=w641) -> (x .and. y?=w640:bool)
              n475 = Select(t=FALSE, s=w640, f=w639) -> (s? t:f=w638:bool)
            }
            frame Disabled {
            }
          }
          n476 = case shown="False" w626 {
            tunnel: w624 -> [_ w689]
            tunnel: w625 -> [_ w688]
            tunnel: [0.5 w687] -> w627
            frame False {
              n477 = local read "Coeff right"() -> (w657:dbl[])
              n478 = local read "Coeff left"() -> (w658:dbl[])
              n479 = Empty Array?(array=w657) -> (empty?=w656:bool)
              n480 = Empty Array?(array=w658) -> (empty?=w654:bool)
              n481 = Exclusive Or(1:w656, 2:w654) -> (0:w655:bool)
              n482 = case shown="False" w655 {
                tunnel: w654 -> [w659 w668]
                frame False {
                  n483 = case shown="True" w659 {
                    frame False {
                      w660 = 0.5
                      n484 = local read "Coeff right"() -> (w664:dbl[])
                      n485 = local read "Coeff left"() -> (w666:dbl[])
                      n486 = Decrement(x=w660) -> (x-1=w665:dbl)
                      n487 = Multiply(x=w666, y=w660) -> (x*y=w663:dbl[])
                      n488 = Multiply(x=w665, y=w664) -> (x*y=w662:dbl[])
                      n489 = Subtract(x=w663, y=w662) -> (x-y=w661:dbl[])
                      n490 = global write "G_SEN.vi" "Lane_C_M"(w661) -> ()
                    }
                    frame True {
                      n491 = local read "Coeff left"() -> (w667:dbl[])
                      n492 = global write "G_SEN.vi" "Lane_C_M"(w667) -> ()
                    }
                  }
                }
                frame True {
                  n493 = case shown="False" w668 {
                    frame False {
                      n494 = global read "G_SEN.vi" "vision lane width"() -> (w671:dbl)
                      n495 = local read "Coeff left"() -> (w677:dbl[])
                      n496 = Index Array(array=w677, index=0) -> (element=w675:dbl)
                      n497 = Multiply(x=w671, y=0.5) -> (x*y=w669:dbl)
                      n498 = Add(x=w675, y=w669) -> (x+y=w674:dbl)
                      n499 = Replace Array Subset(array=w677, new element=w674, index=0) -> (w672:dbl[])
                      n500 = global write "G_SEN.vi" "Lane_C_M"(w672) -> ()
                    }
                    frame True {
                      n501 = global read "G_SEN.vi" "vision lane width"() -> (w680:dbl)
                      n502 = local read "Coeff right"() -> (w686:dbl[])
                      n503 = Index Array(array=w686, index=0) -> (element=w684:dbl)
                      n504 = Multiply(x=w680, y=0.5) -> (x*y=w678:dbl)
                      n505 = Subtract(x=w684, y=w678) -> (x-y=w683:dbl)
                      n506 = Replace Array Subset(array=w686, new element=w683, index=0) -> (w681:dbl[])
                      n507 = global write "G_SEN.vi" "Lane_C_M"(w681) -> ()
                    }
                  }
                }
              }
            }
            frame True {
              n508 = disable-structure shown="Enabled" {
                disable-tunnel: w689 -> [w698 w922]
                disable-tunnel: w688 -> [w697 w921]
                disable-tunnel: [_ w849] -> w687
                frame Disabled {
                  n509 = Absolute Value(x=w698) -> (abs(x)=w720:dbl)
                  n510 = Absolute Value(x=w697) -> (abs(x)=w719:dbl)
                  n511 = global read "G_ALL.vi" "CARSPEC"() -> (w715:T1)
                  n512 = global read "G_ALL.vi" "CARSPEC"() -> (w736:T1)
                  n513 = Build Array(w720, w719) -> (w718:dbl[])
                  n514 = Unbundle By Name(w715) -> ("af"=w714:dbl, "Overall width"=w704:dbl)
                  n515 = Unbundle By Name(w736) -> ("Overall width"=w725:dbl, "af"=w733:dbl, "Overall width"=w721:dbl)
                  n516 = Array Max & Min(array=w718) -> (min value=w711:dbl, min index (indices)=w717:i32)  [unwired: 2 out]
                  n517 = Add(x=w711, y=w725) -> (x+y=w735:dbl)
                  n518 = Square(x=w711) -> (x^2=w702:dbl)
                  n519 = Square(x=w714) -> (x^2=w701:dbl)
                  n520 = Multiply(x=w704, y=0.5) -> (x*y=w703:dbl)
                  n521 = Square(x=w735) -> (x^2=w734:dbl)
                  n522 = Square(x=w733) -> (x^2=w726:dbl)
                  n523 = Subtract(x=w702, y=w701) -> (x-y=w696:dbl)
                  n524 = Multiply(x=w721, y=0.5) -> (x*y=w722:dbl)
                  n525 = Add(x=w734, y=w726) -> (x+y=w732:dbl)
                  n526 = Square Root(x=w696) -> (sqrt(x)=w713:dbl)
                  n527 = global read "G_SEN.vi" "vision lane width"() -> (w707:dbl)
                  n528 = global read "G_SEN.vi" "vision lane width"() -> (w731:dbl)
                  n529 = Subtract(x=w713, y=w704) -> (x-y=w712:dbl)
                  n530 = Square Root(x=w732) -> (sqrt(x)=w730:dbl)
                  n531 = Subtract(x=w711, y=w712) -> (x-y=w706:dbl)
                  n532 = Subtract(x=w730, y=w711) -> (x-y=w729:dbl)
                  n533 = Subtract(x=w707, y=w706) -> (x-y=w708:dbl)
                  n534 = Subtract(x=w731, y=w729) -> (x-y=w728:dbl)
                  n535 = global read "G_SEN.vi" "vision lane width"() -> (w692:dbl)
                  n536 = global read "G_SEN.vi" "vision lane width"() -> (w699:dbl)
                  n537 = Multiply(x=w708, y=0.5) -> (x*y=w710:dbl)
                  n538 = Multiply(x=w728, y=0.5) -> (x*y=w723:dbl)
                  n539 = Compound Arithmetic op=ADD(w710, w703) -> (w700:dbl)
                  n540 = Compound Arithmetic op=ADD(w723, w722) -> (w716:dbl)
                  n541 = Subtract(x=w699, y=w700) -> (x-y=w694:dbl)
                  n542 = Less Than 0?(x=w696) -> (x < 0?=w695:bool)
                  n543 = Multiply(x=0.5 ("y"), y=w692) -> (x*y=w691:dbl)
                  n544 = Select(t=w691, s=w695, f=w694) -> (s? t:f=w693:dbl)
                  n545 = case shown="1" w717 {
                    tunnel: w716 -> [w738 w786]
                    tunnel: w693 -> [w737 w784]
                    frame 0, Default {
                      n546 = local read "Rright"() -> (w740:dbl)
                      n547 = Greater Than 0?(x=w740) -> (x > 0?=w739:bool)
                      n548 = case shown="True" w739 {
                        tunnel: w738 -> [_ w761]
                        tunnel: w737 -> [w743 w760]
                        frame False {
                          n549 = local read "Coeff left"() -> (w742:dbl[])
                          n550 = Empty Array?(array=w742) -> (empty?=w741:bool)
                          n551 = case shown="False" w741 {
                            tunnel: w743 -> [w744 w753]
                            frame False {
                              n552 = global read "G_SEN.vi" "vision lane width"() -> (w752:dbl)
                              n553 = Divide(x=w744, y=w752) -> (x/y=w750:dbl)
                              n554 = local read "Coeff right"() -> (w748:dbl[])
                              n555 = local read "Coeff left"() -> (w751:dbl[])
                              n556 = Decrement(x=w750) -> (x-1=w749:dbl)
                              n557 = Multiply(x=w751, y=w750) -> (x*y=w747:dbl[])
                              n558 = Multiply(x=w749, y=w748) -> (x*y=w746:dbl[])
                              n559 = Subtract(x=w747, y=w746) -> (x-y=w745:dbl[])
                              n560 = global write "G_SEN.vi" "Lane_C_M"(w745) -> ()
                            }
                            frame True {
                              n561 = local read "Coeff right"() -> (w759:dbl[])
                              n562 = Index Array(array=w759, index=0) -> (element=w757:dbl)
                              n563 = Subtract(x=w757, y=w753) -> (x-y=w756:dbl)
                              n564 = Replace Array Subset(array=w759, new element=w756, index=0) -> (w754:dbl[])
                              n565 = global write "G_SEN.vi" "Lane_C_M"(w754) -> ()
                            }
                          }
                        }
                        frame True {
                          n566 = local read "Coeff left"() -> (w763:dbl[])
                          n567 = Empty Array?(array=w763) -> (empty?=w762:bool)
                          n568 = case shown="False" w762 {
                            tunnel: w761 -> [w767 w777]
                            tunnel: w760 -> [w768 _]
                            frame False {
                              n569 = Add(x=w768, y=w767) -> (x+y=w766:dbl)
                              n570 = global read "G_SEN.vi" "vision lane width"() -> (w776:dbl)
                              n571 = Multiply(x=w766, y=0.5) -> (x*y=w764:dbl)
                              n572 = Divide(x=w764, y=w776) -> (x/y=w774:dbl)
                              n573 = local read "Coeff right"() -> (w772:dbl[])
                              n574 = local read "Coeff left"() -> (w775:dbl[])
                              n575 = Decrement(x=w774) -> (x-1=w773:dbl)
                              n576 = Multiply(x=w775, y=w774) -> (x*y=w771:dbl[])
                              n577 = Multiply(x=w773, y=w772) -> (x*y=w770:dbl[])
                              n578 = Subtract(x=w771, y=w770) -> (x-y=w769:dbl[])
                              n579 = global write "G_SEN.vi" "Lane_C_M"(w769) -> ()
                            }
                            frame True {
                              n580 = local read "Coeff right"() -> (w783:dbl[])
                              n581 = Index Array(array=w783, index=0) -> (element=w781:dbl)
                              n582 = Subtract(x=w781, y=w777) -> (x-y=w780:dbl)
                              n583 = Replace Array Subset(array=w783, new element=w780, index=0) -> (w778:dbl[])
                              n584 = global write "G_SEN.vi" "Lane_C_M"(w778) -> ()
                            }
                          }
                        }
                      }
                    }
                    frame 1 {
                      n585 = local read "Rleft"() -> (w787:dbl)
                      n586 = Less Than 0?(x=w787) -> (x < 0?=w785:bool)
                      n587 = case shown="True" w785 {
                        tunnel: w786 -> [_ w808]
                        tunnel: w784 -> [w790 w807]
                        frame False {
                          n588 = local read "Coeff right"() -> (w789:dbl[])
                          n589 = Empty Array?(array=w789) -> (empty?=w788:bool)
                          n590 = case shown="False" w788 {
                            tunnel: w790 -> [w791 w800]
                            frame False {
                              n591 = global read "G_SEN.vi" "vision lane width"() -> (w799:dbl)
                              n592 = Divide(x=w791, y=w799) -> (x/y=w797:dbl)
                              n593 = local read "Coeff right"() -> (w798:dbl[])
                              n594 = local read "Coeff left"() -> (w795:dbl[])
                              n595 = Decrement(x=w797) -> (x-1=w796:dbl)
                              n596 = Multiply(x=w798, y=w797) -> (x*y=w794:dbl[])
                              n597 = Multiply(x=w796, y=w795) -> (x*y=w793:dbl[])
                              n598 = Subtract(x=w794, y=w793) -> (x-y=w792:dbl[])
                              n599 = global write "G_SEN.vi" "Lane_C_M"(w792) -> ()
                            }
                            frame True {
                              n600 = local read "Coeff left"() -> (w806:dbl[])
                              n601 = Index Array(array=w806, index=0) -> (element=w804:dbl)
                              n602 = Add(x=w804, y=w800) -> (x+y=w803:dbl)
                              n603 = Replace Array Subset(array=w806, new element=w803, index=0) -> (w801:dbl[])
                              n604 = global write "G_SEN.vi" "Lane_C_M"(w801) -> ()
                            }
                          }
                        }
                        frame True {
                          n605 = local read "Coeff right"() -> (w810:dbl[])
                          n606 = Empty Array?(array=w810) -> (empty?=w809:bool)
                          n607 = case shown="False" w809 {
                            tunnel: w808 -> [w812 w824]
                            tunnel: w807 -> [w813 _]
                            frame False {
                              n608 = Add(x=w813, y=w812) -> (x+y=w815:dbl)
                              n609 = global read "G_SEN.vi" "vision lane width"() -> (w823:dbl)
                              n610 = Multiply(x=w815, y=0.5) -> (x*y=w811:dbl)
                              n611 = Divide(x=w811, y=w823) -> (x/y=w821:dbl)
                              n612 = local read "Coeff right"() -> (w822:dbl[])
                              n613 = local read "Coeff left"() -> (w819:dbl[])
                              n614 = Decrement(x=w821) -> (x-1=w820:dbl)
                              n615 = Multiply(x=w822, y=w821) -> (x*y=w818:dbl[])
                              n616 = Multiply(x=w820, y=w819) -> (x*y=w817:dbl[])
                              n617 = Subtract(x=w818, y=w817) -> (x-y=w816:dbl[])
                              n618 = global write "G_SEN.vi" "Lane_C_M"(w816) -> ()
                            }
                            frame True {
                              n619 = local read "Coeff left"() -> (w830:dbl[])
                              n620 = Index Array(array=w830, index=0) -> (element=w828:dbl)
                              n621 = Add(x=w828, y=w824) -> (x+y=w827:dbl)
                              n622 = Replace Array Subset(array=w830, new element=w827, index=0) -> (w825:dbl[])
                              n623 = global write "G_SEN.vi" "Lane_C_M"(w825) -> ()
                            }
                          }
                        }
                      }
                    }
                  }
                }
                frame Enabled {
                  n624 = Build Array(w922, w921) -> (w896:dbl[])
                  n625 = global read "G_ALL.vi" "CARSPEC"() -> (w919:T1)
                  n626 = Absolute Value(x=w896) -> (abs(x)=w920:dbl[])
                  n627 = Unbundle By Name(w919) -> ("Overall width"=w918:dbl, "af"=w916:dbl, "Overall width"=w844:dbl)
                  n628 = Array Max & Min(array=w920) -> (max value=w898:dbl, min value=w854:dbl, min index (indices)=w895:i32)  [unwired: 1 out]
                  n629 = global read "G_ALL.vi" "CARSPEC"() -> (w907:T1)
                  n630 = Index Array(array=w896, index=w895) -> (element=w894:dbl)
                  n631 = Add(x=w854, y=w918) -> (x+y=w917:dbl)
                  n632 = Not Equal?(x=inf, y=w898) -> (x != y?=w893:bool)
                  n633 = Multiply(x=w844, y=0.5) -> (x*y=w843:dbl)
                  n634 = Unbundle By Name(w907) -> ("Overall width"=w838:dbl, "af"=w906:dbl)
                  n635 = Select(t=w898, s=w893, f=w854) -> (s? t:f=w897:dbl)
                  n636 = Square(x=w917) -> (x^2=w915:dbl)
                  n637 = Square(x=w916) -> (x^2=w914:dbl)
                  n638 = Square(x=w897) -> (x^2=w904:dbl)
                  n639 = Square(x=w906) -> (x^2=w905:dbl)
                  n640 = Add(x=w915, y=w914) -> (x+y=w913:dbl)
                  n641 = global read "G_SEN.vi" "vision lane width"() -> (w910:dbl)
                  n642 = Subtract(x=w904, y=w905) -> (x-y=w855:dbl)
                  n643 = Square Root(x=w913) -> (sqrt(x)=w912:dbl)
                  n644 = Multiply(x=0.5, y=w838) -> (x*y=w835:dbl)
                  n645 = Subtract(x=w854, y=w912) -> (x-y=w911:dbl)
                  n646 = Max & Min(x=w855, y=w854) -> (max(x,y)=w853:dbl)  [unwired: 1 out]
                  n647 = global read "G_SEN.vi" "vision lane width"() -> (w902:dbl)
                  n648 = Compound Arithmetic op=ADD(w911, w844, w910) -> (w909:dbl)
                  n649 = Square Root(x=w853) -> (sqrt(x)=w903:dbl)
                  n650 = Add(x=w843, y=0.1) -> (x+y=w840:dbl)
                  n651 = Subtract(x=w897, y=w903) -> (x-y=w836:dbl)
                  n652 = Multiply(x=w909, y=0.5) -> (x*y=w841:dbl)
                  n653 = Max & Min(x=w841, y=w840) -> (max(x,y)=w839:dbl)  [unwired: 1 out]
                  n654 = Compound Arithmetic op=ADD(w836, w902) -> (w900:dbl)
                  n655 = Compound Arithmetic op=ADD(0.1 ("value"), w835, w836) -> (w832:dbl)
                  n656 = Multiply(x=w900, y=0.5) -> (x*y=w833:dbl)
                  n657 = Max & Min(x=w832, y=w833) -> (max(x,y)=w831:dbl)  [unwired: 1 out]
                  n658 = case shown="True" w893 {
                    tunnel: w895 -> [w927 w945]
                    tunnel: w894 -> [w926 _]
                    tunnel: w839 -> [w925 w948]
                    tunnel: [w924 w940] -> w892
                    tunnel: w831 -> [w923 w950]
                    frame False {
                      n659 = case shown="1" w927 {
                        tunnel: w926 -> [w932 w939]
                        tunnel: w925 -> [w929 w937]
                        tunnel: [w928 w933] -> w924
                        tunnel: w923 -> [w930 w936]
                        frame 0, Default {
                          n660 = Less Than 0?(x=w932) -> (x < 0?=w931:bool)
                          n661 = Select(t=w930, s=w931, f=w929) -> (s? t:f=w928:dbl)
                        }
                        frame 1 {
                          n662 = Greater Than 0?(x=w939) -> (x > 0?=w938:bool)
                          n663 = global read "G_SEN.vi" "vision lane width"() -> (w935:dbl)
                          n664 = Select(t=w936, s=w938, f=w937) -> (s? t:f=w934:dbl)
                          n665 = Subtract(x=w935, y=w934) -> (x-y=w933:dbl)
                        }
                      }
                    }
                    frame True {
                      n666 = Equal To 0?(x=w945) -> (x = 0?=w944:bool)
                      n667 = global read "G_SEN.vi" "vision lane width"() -> (w951:dbl)
                      n668 = Subtract(x=w951, y=w950) -> (x-y=w949:dbl)
                      n669 = global read "G_SEN.vi" "vision lane width"() -> (w943:dbl)
                      n670 = Add(x=w949, y=w948) -> (x+y=w946:dbl)
                      n671 = Multiply(x=w946, y=0.5) -> (x*y=w942:dbl)
                      n672 = Subtract(x=w943, y=w942) -> (x-y=w941:dbl)
                      n673 = Select(t=w942, s=w944, f=w941) -> (s? t:f=w940:dbl)
                    }
                  }
                  n674 = global read "G_SEN.vi" "vision lane width"() -> (w891:dbl)
                  n675 = local read "Coeff right"() -> (w877:dbl[])
                  n676 = local read "Coeff left"() -> (w864:dbl[])
                  n677 = global read "G_SEN.vi" "vision lane width"() -> (w875:dbl)
                  n678 = global read "G_SEN.vi" "vision lane width"() -> (w866:dbl)
                  n679 = Divide(x=w892, y=w891) -> (x/y=w851:dbl)
                  n680 = local read "poly"() -> (w882:i32)
                  n681 = local read "poly"() -> (w860:i32)
                  n682 = Increment(x=w882) -> (x+1=w881:i32)
                  n683 = Increment(x=w860) -> (x+1=w861:i32)
                  n684 = Index Array(array=w877, index #1=0 ("index")) -> (element #1=w876:dbl, element #2=w857:dbl)  [unwired: 1 in]
                  n685 = Index Array(array=w864, index #1=0 ("index")) -> (element #1=w865:dbl, element #2=w856:dbl)  [unwired: 1 in]
                  n686 = Subtract(x=0.5, y=w851) -> (x-y=w848:dbl)
                  n687 = local read "Coeff right"() -> (w870:dbl[])
                  n688 = Subtract(x=w876, y=w875) -> (x-y=w874:dbl)
                  n689 = Add(x=w865, y=w866) -> (x+y=w867:dbl)
                  n690 = Initialize Array(0.0 ("element"), w881) -> (w880:dbl[])
                  n691 = Initialize Array(0.0 ("element"), w861) -> (w862:dbl[])
                  n692 = local read "Coeff left"() -> (w885:dbl[])
                  n693 = Multiply(x=w848, y="lane_gain") -> (x*y=w847:dbl)
                  n694 = Empty Array?(array=w870) -> (empty?=w872:bool)
                  n695 = Empty Array?(array=w885) -> (empty?=w886:bool)
                  n696 = Replace Array Subset(array=w880, new element #1=w874, index #1=0 ("index"), new element #2=w857) -> (w879:dbl[])  [unwired: 1 in]
                  n697 = Replace Array Subset(array=w862, new element #1=w867, index #1=0 ("index"), new element #2=w856) -> (w858:dbl[])  [unwired: 1 in]
                  n698 = Not(x=w872) -> (.not. x?=w871:bool)
                  n699 = Subtract(x=0.5 ("y"), y=w847) -> (x-y=w849:dbl)
                  n700 = Select(t=w879, s=w886, f=w885) -> (s? t:f=w884:dbl[])
                  n701 = Select(t=w870, s=w871, f=w858) -> (s? t:f=w869:dbl[])
                  n702 = Decrement(x=w849) -> (x-1=w890:dbl)
                  n703 = Multiply(x=w884, y=w849) -> (x*y=w888:dbl[])
                  n704 = Multiply(x=w890, y=w869) -> (x*y=w889:dbl[])
                  n705 = Subtract(x=w888, y=w889) -> (x-y=w887:dbl[])
                  n706 = global write "G_SEN.vi" "Lane_C_M"(w887) -> ()
                }
              }
            }
          }
          n707 = Subtract(x=0.5, y=w627) -> (x-y=w629:dbl)
          n708 = Multiply(x=w629, y=2.0) -> (x*y=→"ratio(-1:left1:right)":dbl)
        }
        frame #2 {
          n709 = global read "G_SEN.vi" "Lane_C_M"() -> (w952:dbl[])
          "Lane_C_M" <- w952
          n710 = Index Array(array=w952, index=0) -> (element=w954:dbl)
          n711 = Not A Number/Path/Refnum?(number/path/refnum=w954) -> (NaN/Path/Refnum?=w955:bool)
          n712 = case shown="True" w955 {
            selector: w955 -> [_ w956]
            frame False {
            }
            frame True {
              "NaN/Path/Refnum?" <- w956
            }
          }
        }
      }
    }
    frame #3 {
      n713 = global read "G_ALL.vi" "map_track 2"() -> (w959:dbl[][])
      n714 = Empty Array?(array=w959) -> (empty?=w957:bool)
      n715 = case shown="False" w957 {
        tunnel: [w967 _] -> w960
        tunnel: [w966 _] -> w961
        tunnel: [w965 _] -> w958
        tunnel: w959 -> [w964 _]
        frame False {
          n716 = flat-sequence {
            tunnel: w964 -> [w968]
            tunnel: [w1083] -> w967
            tunnel: [w1082] -> w966
            tunnel: [w1081] -> w965
            frame #0 {
              n717 = global read "G_ALL.vi" "dist"() -> (w973:dbl[])
              n718 = Threshold 1D Array(2:-4.0 ("threshold y"), 3:w973) -> (0:w971:dbl)  [unwired: 1 in]
              n719 = Round Toward +Infinity(x=w971) -> (ceil(x): smallest int >= x=w969:dbl)
              n720 = Array Subset(array=w968, index (row)=w969) -> (→"map_track":dbl[][])  [unwired: 3 in]
            }
            frame #1 {
              n721 = local read "d_safe"() -> (w980:dbl)
              n722 = local read "y 2"() -> (w977:dbl[])
              n723 = Array Size(array=w977) -> (size(s)=w976:i32)
              n724 = Subtract(x=w980, y=0.2) -> (x-y=w979:dbl)
              n725 = local read "map_track"() -> (w974:dbl[][])
              n726 = local read "x 2"() -> (w981:dbl[])
              n727 = for {
                N: w976 -> [_]
                tunnel: w977 -> [w989] mode=indexing
                tunnel: w981 -> [w990] mode=indexing
                tunnel: w974 -> [w995]
                tunnel: w979 -> [w991]
                tunnel: [w987] -> w982 mode=indexing
                tunnel: [w984] -> w975 mode=indexing
                i -> [w985]
                n728 = Build Array(w990, w989) -> (w988:dbl[])
                n729 = Index Array(array=w995, index (col) #1=0 ("disabled index (col)")) -> (element #1=w1003:dbl[], element #2=w1002:dbl[])  [unwired: 3 in]
                n730 = Subtract(x=w990, y=w1003) -> (x-y=w1000:dbl[])
                n731 = Subtract(x=w1002, y=w989) -> (x-y=w1001:dbl[])
                n732 = Square(x=w1000) -> (x^2=w999:dbl[])
                n733 = Square(x=w1001) -> (x^2=w998:dbl[])
                n734 = Add(x=w999, y=w998) -> (x+y=w997:dbl[])
                n735 = Square Root(x=w997) -> (sqrt(x)=w996:dbl[])
                n736 = Array Max & Min(array=w996) -> (min value=w992:dbl, min index (indices)=w994:i32)  [unwired: 2 out]
                n737 = Less Or Equal?(x=w991, y=w992) -> (x <= y?=w993:bool)
                n738 = case shown="True" w993 {
                  tunnel: w995 -> [_ w1026]
                  tunnel: w994 -> [_ w1025]
                  tunnel: w988 -> [_ w1019]
                  tunnel: [_ w1007] -> w987
                  frame False {
                  }
                  frame True {
                    n739 = Decrement(x=w1025) -> (x-1=w1024:i32)
                    n740 = Max & Min(x=w1024, y=0) -> (max(x,y)=w1023:i32)  [unwired: 1 out]
                    n741 = Index Array(array=w1026, index (row) #1=w1023) -> (element #1=w1020:dbl[], element #2=w1021:dbl[])  [unwired: 3 in]
                    n742 = Subtract(x=w1019, y=w1020) -> (x-y=w1016:dbl[])
                    n743 = Subtract(x=w1021, y=w1020) -> (x-y=w1018:dbl[])
                    n744 = Index Array(array=w1016, index #1=0 ("index"), index #2=1 ("index")) -> (element #1=w1010:dbl, element #2=w1012:dbl)
                    n745 = Index Array(array=w1018, index #1=0 ("index"), index #2=1 ("index")) -> (element #1=w1011:dbl, element #2=w1009:dbl)
                    n746 = Multiply(x=w1010, y=w1009) -> (x*y=w1006:dbl)
                    n747 = Multiply(x=w1012, y=w1011) -> (x*y=w1005:dbl)
                    n748 = Subtract(x=w1006, y=w1005) -> (x-y=w1008:dbl)
                    n749 = Sign(1:w1008) -> (0:w1007:dbl)
                  }
                }
                n750 = local read "w"() -> (w986:dbl[])
                n751 = Index Array(array=w986, index=w985) -> (element=w984:dbl)
              }
              "w 2" <- w982
              n752 = disable-structure shown="Disabled" {
                disable-tunnel: w975 -> [w983 _]
                frame Disabled {
                  n753 = local write "w"(w983) -> ()
                }
                frame Enabled {
                }
              }
            }
            frame #2 {
              n754 = local read "w"() -> (w1042:dbl[])
              n755 = local read "w"() -> (w1043:dbl[])
              n756 = Greater Or Equal?(x=w1042, y=1.0) -> (x >= y?=w1028:bool[])
              n757 = Less Or Equal?(x=w1043, y=-1.0) -> (x <= y?=w1027:bool[])
              n758 = local read "y"() -> (w1050:dbl[])
              n759 = local read "y"() -> (w1071:dbl[])
              n760 = local read "x"() -> (w1049:dbl[])
              n761 = local read "x"() -> (w1072:dbl[])
              n762 = local read "w"() -> (w1045:dbl[])
              n763 = local read "w"() -> (w1037:dbl[])
              n764 = local read "w"() -> (w1048:dbl[])
              n765 = local read "w"() -> (w1034:dbl[])
              n766 = Boolean To (0,1)(Boolean=w1028) -> (0, 1=w1055:i16[])
              n767 = Boolean To (0,1)(Boolean=w1027) -> (0, 1=w1066:i16[])
              n768 = Build Cluster Array(w1028, w1049, w1050) -> (w1051:cluster{bool, dbl, dbl}[])
              n769 = Build Cluster Array(w1027, w1072, w1071) -> (w1070:cluster{bool, dbl, dbl}[])
              n770 = Greater Or Equal?(x=w1045, y=1.0) -> (x >= y?=w1039:bool[])
              n771 = Less Or Equal?(x=w1037, y=-1.0) -> (x <= y?=w1036:bool[])
              n772 = Less Or Equal?(x=w1048, y=-1.0) -> (x <= y?=w1040:bool[])
              n773 = Greater Or Equal?(x=w1034, y=1.0) -> (x >= y?=w1032:bool[])
              n774 = Or(x=w1039, y=w1028) -> (x .or. y?=w1029:bool[])
              n775 = Or(x=w1040, y=w1027) -> (x .or. y?=w1030:bool[])
              n776 = To Long Integer(number=w1055) -> (32bit integer=w1056:i32[])
              n777 = Not(x=w1036) -> (.not. x?=w1035:bool[])
              n778 = Not(x=w1032) -> (.not. x?=w1031:bool[])
              n779 = To Long Integer(number=w1066) -> (32bit integer=w1065:i32[])
              n780 = Sort 1D Array(array=w1051) -> (sorted array=w1052:cluster{bool, dbl, dbl}[])
              n781 = Sort 1D Array(array=w1070) -> (sorted array=w1069:cluster{bool, dbl, dbl}[])
              n782 = And(x=w1029, y=w1035) -> ()  [unwired: 1 out]
              n783 = And(x=w1030, y=w1031) -> ()  [unwired: 1 out]
              n784 = Add Array Elements(numeric array=w1056) -> (sum=w1054:i32)
              n785 = Add Array Elements(numeric array=w1065) -> (sum=w1067:i32)
              n786 = Reverse 1D Array(array=w1052) -> (reversed array=w1053:cluster{bool, dbl, dbl}[])
              n787 = Reverse 1D Array(array=w1069) -> (reversed array=w1068:cluster{bool, dbl, dbl}[])
              n788 = for {
                N: w1054 -> [_]
                tunnel: w1053 -> [w1076] mode=indexing
                tunnel: [w1075] -> w1058 mode=indexing
                tunnel: [w1074] -> w1057 mode=indexing
                tunnel: [w1073] -> _
                i -> [w1073]
                n789 = Unbundle(w1076) -> (w1075:dbl, w1074:dbl)  [unwired: 1 out]
              }
              n790 = for {
                N: w1067 -> [_]
                tunnel: w1068 -> [w1080] mode=indexing
                tunnel: [w1079] -> w1063 mode=indexing
                tunnel: [w1078] -> w1064 mode=indexing
                tunnel: [w1077] -> _
                i -> [w1077]
                n791 = Unbundle(w1080) -> (w1079:dbl, w1078:dbl)  [unwired: 1 out]
              }
              n792 = Build Array(w1058, w1057) -> (w1059:dbl[][])
              n793 = Build Array(w1063, w1064) -> (w1062:dbl[][])
              n794 = Transpose 2D Array(2D array=w1059) -> (transposed array=→"lane_right_pt":dbl[][])
              n795 = Transpose 2D Array(2D array=w1062) -> (transposed array=→"lane_left_pt":dbl[][])
            }
            frame #3 {
              n796 = local read "lane_right_pt"() -> (w1107:dbl[][])
              n797 = local read "lane_left_pt"() -> (w1105:dbl[][])
              n798 = Empty Array?(array=w1107) -> (empty?=w1106:bool)
              n799 = Empty Array?(array=w1105) -> (empty?=w1104:bool)
              n800 = case shown="False" w1106 {
                tunnel: [w1159 _] -> w1101
                tunnel: [w1158 _] -> w1098
                frame False {
                  n801 = local read "lane_right_pt"() -> (w1161:dbl[][])
                  n802 = local read "map_track"() -> (w1165:dbl[][])
                  n803 = Index Array(array=w1161, index (col) #1=0 ("disabled index (col)")) -> (element #1=w1163:dbl[], element #2=w1164:dbl[])  [unwired: 3 in]
                  n804 = Delete From Array(array=w1165, index (row)=0) -> (deleted portion=w1168:dbl[], array with subset deleted=w1166:dbl[][])  [unwired: 2 in]
                  n805 = local read "d_safe"() -> (w1160:dbl)
                  n806 = for {
                    tunnel: w1163 -> [w1200]
                    tunnel: w1164 -> [w1199]
                    tunnel: w1166 -> [w1190] mode=indexing
                    shift-right: [w1190] -> _
                    shift-left: w1168 -> [w1189]
                    tunnel: [w1178] -> w1169 mode=indexing
                    tunnel: [w1176] -> w1170 mode=indexing
                    tunnel: w1160 -> [w1177]
                    n807 = Subtract(x=w1190, y=w1189) -> (x-y=w1188:dbl[])
                    n808 = Index Array(array=w1190) -> (element #1=w1192:dbl, element #2=w1191:dbl)  [unwired: 2 in]
                    n809 = Subtract(x=w1200, y=w1192) -> (x-y=w1198:dbl[])
                    n810 = Subtract(x=w1199, y=w1191) -> (x-y=w1197:dbl[])
                    n811 = Index Array(array=w1188, index #1=1 ("index"), index #2=0 ("index")) -> (element #1=w1185:dbl, element #2=w1184:dbl)
                    n812 = Square(x=w1198) -> (x^2=w1195:dbl[])
                    n813 = Square(x=w1197) -> (x^2=w1196:dbl[])
                    n814 = Inverse Tangent (2 Input)(1:w1184, 2:w1185) -> (0:w1183:dbl)
                    n815 = Add(x=w1195, y=w1196) -> (x+y=w1194:dbl[])
                    n816 = call "headingoperater.vi"("h1"=1.5707963267948966, "h2"=w1183) -> ("h2+h1"=w1176:dbl)  [unwired: 8 in, 1 out]
                    n817 = Square Root(x=w1194) -> (sqrt(x)=w1193:dbl[])
                    n818 = Array Max & Min(array=w1193) -> (min value=w1181:dbl)  [unwired: 3 out]
                    n819 = Subtract(x=w1177, y=w1181) -> (x-y=w1180:dbl)
                    n820 = Max & Min(x=w1180, y=0.0) -> (max(x,y)=w1178:dbl)  [unwired: 1 out]
                  }
                  n821 = Polar To Re/Im(2:w1170, 3:w1169) -> (0:w1172:dbl[], 1:w1171:dbl[])
                  n822 = Add Array Elements(numeric array=w1171) -> (sum=w1174:dbl)
                  n823 = Add Array Elements(numeric array=w1172) -> (sum=w1173:dbl)
                  n824 = Array Size(array=w1172) -> (size(s)=w1175:i32)
                  n825 = Divide(x=w1174, y=w1175) -> (x/y=w1159:dbl)
                  n826 = Divide(x=w1173, y=w1175) -> (x/y=w1158:dbl)
                }
                frame True {
                }
              }
              n827 = case shown="False" w1104 {
                tunnel: [w1116 _] -> w1092
                tunnel: [w1115 _] -> w1095
                frame False {
                  n828 = local read "lane_left_pt"() -> (w1132:dbl[][])
                  n829 = local read "map_track"() -> (w1128:dbl[][])
                  n830 = Index Array(array=w1132, index (col) #1=0 ("disabled index (col)")) -> (element #1=w1130:dbl[], element #2=w1129:dbl[])  [unwired: 3 in]
                  n831 = Delete From Array(array=w1128, index (row)=0) -> (deleted portion=w1125:dbl[], array with subset deleted=w1127:dbl[][])  [unwired: 2 in]
                  n832 = local read "d_safe"() -> (w1117:dbl)
                  n833 = for {
                    tunnel: w1130 -> [w1157]
                    tunnel: w1129 -> [w1156]
                    tunnel: w1127 -> [w1147] mode=indexing
                    shift-right: [w1147] -> _
                    shift-left: w1125 -> [w1146]
                    tunnel: [w1134] -> w1124 mode=indexing
                    tunnel: [w1135] -> w1123 mode=indexing
                    tunnel: w1117 -> [w1133]
                    n834 = Subtract(x=w1147, y=w1146) -> (x-y=w1145:dbl[])
                    n835 = Index Array(array=w1147) -> (element #1=w1149:dbl, element #2=w1148:dbl)  [unwired: 2 in]
                    n836 = Subtract(x=w1157, y=w1149) -> (x-y=w1155:dbl[])
                    n837 = Subtract(x=w1156, y=w1148) -> (x-y=w1154:dbl[])
                    n838 = Index Array(array=w1145, index #1=1 ("index"), index #2=0 ("index")) -> (element #1=w1142:dbl, element #2=w1141:dbl)
                    n839 = Square(x=w1155) -> (x^2=w1152:dbl[])
                    n840 = Square(x=w1154) -> (x^2=w1153:dbl[])
                    n841 = Inverse Tangent (2 Input)(1:w1141, 2:w1142) -> (0:w1140:dbl)
                    n842 = Add(x=w1152, y=w1153) -> (x+y=w1151:dbl[])
                    n843 = call "headingoperater.vi"("h1"=1.5707963267948966, "h2"=w1140) -> ("h2-h1"=w1135:dbl)  [unwired: 8 in, 1 out]
                    n844 = Square Root(x=w1151) -> (sqrt(x)=w1150:dbl[])
                    n845 = Array Max & Min(array=w1150) -> (min value=w1138:dbl)  [unwired: 3 out]
                    n846 = Subtract(x=w1133, y=w1138) -> (x-y=w1137:dbl)
                    n847 = Max & Min(x=w1137, y=0.0) -> (max(x,y)=w1134:dbl)  [unwired: 1 out]
                  }
                  n848 = Polar To Re/Im(2:w1123, 3:w1124) -> (0:w1121:dbl[], 1:w1122:dbl[])
                  n849 = Add Array Elements(numeric array=w1122) -> (sum=w1119:dbl)
                  n850 = Add Array Elements(numeric array=w1121) -> (sum=w1120:dbl)
                  n851 = Array Size(array=w1121) -> (size(s)=w1118:i32)
                  n852 = Divide(x=w1119, y=w1118) -> (x/y=w1116:dbl)
                  n853 = Divide(x=w1120, y=w1118) -> (x/y=w1115:dbl)
                }
                frame True {
                }
              }
              n854 = Not A Number/Path/Refnum?(number/path/refnum=w1101) -> (NaN/Path/Refnum?=w1103:bool)
              n855 = Not A Number/Path/Refnum?(number/path/refnum=w1092) -> (NaN/Path/Refnum?=w1093:bool)
              n856 = Not A Number/Path/Refnum?(number/path/refnum=w1098) -> (NaN/Path/Refnum?=w1099:bool)
              n857 = Not A Number/Path/Refnum?(number/path/refnum=w1095) -> (NaN/Path/Refnum?=w1097:bool)
              n858 = local read "map_track"() -> (w1114:dbl[][])
              n859 = Select(t=0.0, s=w1103, f=w1101) -> (s? t:f=w1089:dbl)
              n860 = Select(t=0.0, s=w1093, f=w1092) -> (s? t:f=w1088:dbl)
              n861 = Select(t=0.0, s=w1099, f=w1098) -> (s? t:f=w1086:dbl)
              n862 = Select(t=0.0, s=w1097, f=w1095) -> (s? t:f=w1087:dbl)
              n863 = Add(x=w1089, y=w1088) -> (x+y=w1090:dbl)
              n864 = Add(x=w1086, y=w1087) -> (x+y=w1084:dbl)
              n865 = Index Array(array=w1114, index (col) #1=0 ("disabled index (col)")) -> (element #1=w1112:dbl[], element #2=w1111:dbl[])  [unwired: 3 in]
              n866 = Add(x=w1090, y=w1112) -> (x+y=w1110:dbl[])
              n867 = Add(x=w1084, y=w1111) -> (x+y=w1109:dbl[])
              n868 = Multiply(x="x_gain", y=w1090) -> (x*y=w1083:dbl)
              n869 = Multiply(x=w1084, y="y_gain") -> (x*y=w1082:dbl)
              n870 = Build Array(w1110, w1109) -> (w1108:dbl[][])
              n871 = Transpose 2D Array(2D array=w1108) -> (transposed array=w1081:dbl[][])
            }
          }
        }
        frame True {
        }
      }
      "map_track 2" <- w958
      "y_shift" <- w961
      "x_shift" <- w960
      n872 = disable-structure shown="Disabled" {
        disable-tunnel: w961 -> [w963 _]
        disable-tunnel: w960 -> [w962 _]
        frame Disabled {
          n873 = global write "G_SEN.vi" "vision x shift"(w962) -> ()
          n874 = global write "G_SEN.vi" "vision y shift"(w963) -> ()
        }
        frame Enabled {
        }
      }
    }
    frame #4 {
      n875 = disable-structure shown="Enabled" {
        frame Enabled {
          n876 = local read "w"() -> (w1308:dbl[])
          n877 = local read "w"() -> (w1290:dbl[])
          n878 = local read "w 2"() -> (w1220:dbl[])
          n879 = local read "w 2"() -> (w1221:dbl[])
          n880 = local read "w"() -> (→"Waveform Graph":dbl[])
          n881 = Less Or Equal?(x=w1308, y=-1.0) -> (x <= y?=w1201:bool[])
          n882 = Greater Or Equal?(x=w1290, y=1.0) -> (x >= y?=w1202:bool[])
          n883 = local read "y"() -> (w1305:dbl[])
          n884 = local read "y"() -> (w1293:dbl[])
          n885 = local read "x"() -> (w1306:dbl[])
          n886 = local read "x"() -> (w1292:dbl[])
          n887 = local read "w"() -> (w1215:dbl[])
          n888 = local read "w"() -> (w1212:dbl[])
          n889 = Greater Or Equal?(x=w1220, y=1.0) -> (x >= y?=w1217:bool[])
          n890 = Less Or Equal?(x=w1221, y=-1.0) -> (x <= y?=w1218:bool[])
          n891 = Build Cluster Array(w1201, w1306, w1305) -> (w1304:cluster{bool, dbl, dbl}[])
          n892 = Build Cluster Array(w1202, w1292, w1293) -> (w1294:cluster{bool, dbl, dbl}[])
          n893 = Less Or Equal?(x=w1215, y=-1.0) -> (x <= y?=w1214:bool[])
          n894 = Greater Or Equal?(x=w1212, y=1.0) -> (x >= y?=w1210:bool[])
          n895 = Or(x=w1202, y=w1217) -> (x .or. y?=w1207:bool[])
          n896 = Or(x=w1201, y=w1218) -> (x .or. y?=w1208:bool[])
          n897 = Not(x=w1214) -> (.not. x?=w1213:bool[])
          n898 = Not(x=w1210) -> (.not. x?=w1209:bool[])
          n899 = Sort 1D Array(array=w1304) -> (sorted array=w1303:cluster{bool, dbl, dbl}[])
          n900 = Sort 1D Array(array=w1294) -> (sorted array=w1295:cluster{bool, dbl, dbl}[])
          n901 = And(x=w1207, y=w1213) -> ()  [unwired: 1 out]
          n902 = And(x=w1208, y=w1209) -> ()  [unwired: 1 out]
          n903 = Reverse 1D Array(array=w1303) -> (reversed array=w1302:cluster{bool, dbl, dbl}[])
          n904 = Reverse 1D Array(array=w1295) -> (reversed array=w1296:cluster{bool, dbl, dbl}[])
          n905 = for {
            tunnel: w1302 -> [w1322] mode=indexing
            tunnel: [w1320] -> w1301 mode=indexing
            tunnel: [w1319] -> w1285 mode=indexing
            tunnel: [w1318] -> w1300
            i -> [w1318]
            stop <- w1321 continue-if-true
            n906 = Unbundle(w1322) -> (w1321:bool, w1320:dbl, w1319:dbl)
          }
          n907 = for {
            tunnel: w1296 -> [w1317] mode=indexing
            tunnel: [w1315] -> w1297 mode=indexing
            tunnel: [w1314] -> w1283 mode=indexing
            tunnel: [w1313] -> w1298
            i -> [w1313]
            stop <- w1316 continue-if-true
            n908 = Unbundle(w1317) -> (w1316:bool, w1315:dbl, w1314:dbl)
          }
          n909 = Array Subset(array=w1301, index=0, length=w1300) -> (w1299:dbl[])
          n910 = Array Subset(array=w1285, index=0, length=w1300) -> (w1282:dbl[])
          n911 = Array Subset(array=w1283, index=0, length=w1298) -> (w1278:dbl[])
          n912 = Array Subset(array=w1297, index=0, length=w1298) -> (w1289:dbl[])
          n913 = local read "map_track"() -> (w1231:dbl[][])
          n914 = call "Convert to Dynamic Data4"("Array"=w1299) -> ("Dynamic Data Type"=w1267:dynamicdata)  [unwired: 3 in]
          n915 = call "Convert to Dynamic Data3"("Array"=w1282) -> ("Dynamic Data Type"=w1279:dynamicdata)  [unwired: 3 in]
          n916 = call "Convert to Dynamic Data6"("Array"=w1289) -> ("Dynamic Data Type"=w1265:dynamicdata)  [unwired: 3 in]
          n917 = call "Convert to Dynamic Data8"("Array"=w1278) -> ("Dynamic Data Type"=w1277:dynamicdata)  [unwired: 3 in]
          n918 = Array Max & Min(array=w1282) -> (max value=w1206:dbl, min value=w1205:dbl)  [unwired: 2 out]
          n919 = Array Max & Min(array=w1278) -> (max value=w1204:dbl, min value=w1203:dbl)  [unwired: 2 out]
          n920 = Add(x=w1206, y=w1204) -> (x+y=w1250:dbl)
          n921 = Add(x=w1205, y=w1203) -> (x+y=w1246:dbl)
          n922 = Index Array(array=w1231, index (col) #1=0 ("disabled index (col)")) -> (element #1=w1233:dbl[], element #2=w1235:dbl[])  [unwired: 3 in]
          n923 = call-poly <vilib>:"Ramp Pattern.vi"("start"=w1205, "end"=w1206, "delta"=0.01) -> ("Ramp Pattern"=w1254:dbl[])  [unwired: 6 in, 2 out]
          n924 = call-poly <vilib>:"Ramp Pattern.vi"("start"=w1203, "end"=w1204, "delta"=0.01) -> ("Ramp Pattern"=w1253:dbl[])  [unwired: 6 in, 2 out]
          n925 = local read "map_track 2"() -> (w1230:dbl[][])
          n926 = local read "Coeff stop 2"() -> (w1288:dbl[])
          n927 = local read "Coeff right"() -> (w1252:dbl[])
          n928 = local read "Coeff left"() -> (w1311:dbl[])
          n929 = local read "x_shift"() -> (w1224:dbl)
          n930 = local read "y_shift"() -> (w1223:dbl)
          n931 = local read "y_end"() -> (w1287:dbl[])
          n932 = call "Convert to Dynamic Data7"("Array"=w1254) -> ("Dynamic Data Type"=w1264:dynamicdata)  [unwired: 3 in]
          n933 = call "Convert to Dynamic Data11"("Array"=w1253) -> ("Dynamic Data Type"=w1263:dynamicdata)  [unwired: 3 in]
          n934 = Multiply(x=w1250, y=0.5) -> (x*y=w1248:dbl)
          n935 = Multiply(x=w1246, y=0.5) -> (x*y=w1245:dbl)
          n936 = call-poly <vilib>:"Polynomial Evaluation.vi"("P(x)"=w1288, "A"=w1287) -> ("P(A)"=w1261:dbl[])  [unwired: 1 out]
          n937 = Add(x=w1233, y=w1224) -> (x+y=w1232:dbl[])
          n938 = Add(x=w1235, y=w1223) -> (x+y=w1234:dbl[])
          n939 = call-poly <vilib>:"Polynomial Evaluation.vi"("P(x)"=w1311, "A"=w1254) -> ("P(A)"=w1260:dbl[])  [unwired: 1 out]
          n940 = call-poly <vilib>:"Polynomial Evaluation.vi"("P(x)"=w1252, "A"=w1253) -> ("P(A)"=w1255:dbl[])  [unwired: 1 out]
          n941 = Index Array(array=w1230, index (col) #1=0 ("disabled index (col)")) -> (element #1=w1228:dbl[], element #2=w1226:dbl[])  [unwired: 3 in]
          n942 = call-poly <vilib>:"Ramp Pattern.vi"("start"=w1245, "end"=w1248, "delta"=0.01) -> ("Ramp Pattern"=w1241:dbl[])  [unwired: 6 in, 2 out]
          n943 = global read "G_SEN.vi" "Lane_C_M"() -> (w1244:dbl[])
          n944 = Build Array(w1260, w1254) -> (w1259:dbl[][])
          n945 = Build Array(w1255, w1253) -> (w1256:dbl[][])
          n946 = call "Convert to Dynamic Data2"("Array"=w1260) -> ("Dynamic Data Type"=w1268:dynamicdata)  [unwired: 3 in]
          n947 = call "Convert to Dynamic Data5"("Array"=w1255) -> ("Dynamic Data Type"=w1266:dynamicdata)  [unwired: 3 in]
          n948 = call "Convert to Dynamic Data15"("Array"=w1232) -> ("Dynamic Data Type"=w1238:dynamicdata)  [unwired: 3 in]
          n949 = call "Convert to Dynamic Data14"("Array"=w1241) -> ("Dynamic Data Type"=w1240:dynamicdata)  [unwired: 3 in]
          n950 = call "Convert to Dynamic Data17"("Array"=w1228) -> ("Dynamic Data Type"=w1227:dynamicdata)  [unwired: 3 in]
          n951 = call "Convert to Dynamic Data18"("Array"=w1226) -> ("Dynamic Data Type"=w1225:dynamicdata)  [unwired: 3 in]
          n952 = call "Convert to Dynamic Data"("Array"=w1261) -> ("Dynamic Data Type"=w1273:dynamicdata)  [unwired: 3 in]
          n953 = call "Convert to Dynamic Data16"("Array"=w1234) -> ("Dynamic Data Type"=w1237:dynamicdata)  [unwired: 3 in]
          n954 = local read "y 2"() -> (w1310:dbl[])
          n955 = call-poly <vilib>:"Polynomial Evaluation.vi"("P(x)"=w1244, "A"=w1241) -> ("P(A)"=w1243:dbl[])  [unwired: 1 out]
          n956 = local read "y_end"() -> (w1262:dbl[])
          n957 = Transpose 2D Array(2D array=w1259) -> (transposed array=w1258:dbl[][])
          n958 = Transpose 2D Array(2D array=w1256) -> (transposed array=w1257:dbl[][])
          n959 = call "Convert to Dynamic Data10"("Array"=w1310) -> ("Dynamic Data Type"=w1275:dynamicdata)  [unwired: 3 in]
          n960 = global write "G_SEN.vi" "Lane_L_V"(w1258) -> ()
          n961 = global write "G_SEN.vi" "Lane_R_V"(w1257) -> ()
          n962 = Merge Signals(w1264, w1279, w1263, w1277, w1275, w1273, w1240, w1237, w1225) -> (w1280:dynamicdata)
          n963 = call "Convert to Dynamic Data12"("Array"=w1262) -> ("Dynamic Data Type"=w1274:dynamicdata)  [unwired: 3 in]
          n964 = call "Convert to Dynamic Data13"("Array"=w1243) -> ("Dynamic Data Type"=w1242:dynamicdata)  [unwired: 3 in]
          n965 = local read "x 2"() -> (w1309:dbl[])
          n966 = call "Convert to Dynamic Data9"("Array"=w1309) -> ("Dynamic Data Type"=w1276:dynamicdata)  [unwired: 3 in]
          n967 = Merge Signals(w1268, w1267, w1266, w1265, w1276, w1274, w1242, w1238, w1227) -> (w1281:dynamicdata)
          n968 = call "Build XY Graph"("Y Input"=w1280, "X Input"=w1281) -> ("XY Graph"=→"XY Graph 4":cluster{"X":dbl[], "Y":dbl[]}[])  [unwired: 8 in, 1 out]
        }
        frame Disabled {
        }
      }
    }
  }
